vi "raptor.vi"(11 "Raptor Parameters":T1={"Vertical Search Range"=20, "Template Width"=180, "Template Height"=100, "Correlation Threshold"=0.5, "Surface Morph Size"=10, "En Face Width"=400, "En Face Height"=600, "En Face Depth"=15, "Aspect Ratio"=1.1, "Continous Scan"=FALSE, "Num En Face Reviews"=10, "Fluoresence Channel"=TRUE, "Track Depth"=TRUE, "Auto Expand"=TRUE, "Show Raptor Window"=TRUE, "Surface Threshold"=2, "Gaussian Filter Size"=1.5, "Mean Filter Size"=5.0}) -> ()   [LabVIEW 2016]
doc: "Main vi for Raptor OCT volume assembly system.\nMike Hughes, Applied Optics Group, University of Kent"
uses:
  typedef/raptor_parameters.ctl
  typedef/raptor_state.ctl
  <vilib>/vision/Image Controls.llb/IMAQ Image.ctl
  typedef/build_record.ctl
  typedef/raptor_states.ctl
  typedef/raptor_message.ctl
  typedef/raptor_image.ctl
  globals/Channel 1 Image Ring.vi
  globals/Channel 2 Image Ring.vi
  <vilib>/vision/NI_Vision_Development_Module.lvlib
  <vilib>/Analysis/NI_AALPro.lvlib
panel:
  out "B-scan Processed":i64=1000
  out "Surface Position":cluster{i32[], i32[]}(graph)={[2, 3, 4, 5, 6, 7, 8, 9, 11, 12, 13, 14, 15, 16, 17, 18, 19, 20, 21, 22, 23, 24, 25, 26, 28, 30, 40, 42, 45, 48, 51, 54, 56, 58, 60, 61, 63, 65, 67, 69, 71, 74, 76, 78, 80, 82, 84, 85, 87, 89, 91, 93, 95, 97, 99, 102, 104, 106, 108, 110, 112, 114, 117, 120, 123, 133, 137, 140, 143, 146, 149, 153, 157, 168, 171, 174, 177, 181, 186, 195, 198, 201, 205, 229, 233, 236, 238, 240, 243, 245, 249, 253, 259, 264, 268, 273, 276, 279, 282, 300, 302, 305, 307, 309, 311, 314, 321, 326, 329, 331, 333, 335, 336, 338, 340, 342, 344, 348, 354, 358, 361, 364, 366, 368, 370, 372, 374, 377, 380, 386, 390, 393, 396, 400, 405, 408, 410, 412, 414, 416, 417, 418, 419, 420, 421, 423, 425, 427, 429, 431, 434, 438, 441, 443, 445, 447, 448, 449, 450, 451, 452, 453, 454, 455, 456, 457, 458, 459, 461, 463, 465, 469, 484, 488, 490, 493, 495, 497, 499, 502, 506, 511, 515, 517, 519, 521, 522, 524, 526, 528, 537, 539, 541, 544, 549, 551, 553, 554, 556, 558, 560, 562, 564, 567, 569, 571, 573, 575, 577, 579, 581, 585, 594, 599, 602, 605, 607, 609, 611, 613, 616, 620, 625, 629, 634, 640, 644, 651, 653, 655, 661, 665, 673, 677, 681, 684, 687, 695, 700, 702, 704, 705, 707, 709, 711, 714, 718, 723, 726, 731, 734, 737, 742, 750, 753, 767, 780, 784, 801, 804, 806, 808, 810, 812, 814, 816, 818, 820, 823, 826, 828, 830, 832, 834, 836, 840, 844, 847, 850, 852, 854, 856, 858, 860, 864, 879, 883, 886, 888, 890, 892, 894, 896, 900, 903, 918, 920, 923, 925, 927, 929, 931, 933, 938, 949, 951, 953, 955, 958, 961, 964, 967, 970, 973, 977, 983, 988, 991, 994, 996, 999], [125, 124, 124, 124, 124, 124, 124, 125, 125, 125, 125, 125, 125, 126, 126, 126, 126, 126, 126, 125, 125, 125, 125, 125, 125, 125, 125, 125, 125, 125, 125, 122, 122, 122, 122, 122, 122, 122, 122, 122, 122, 122, 122, 120, 120, 120, 120, 120, 120, 125, 125, 125, 125, 125, 125, 130, 130, 130, 130, 130, 130, 132, 132, 132, 132, 132, 132, 138, 138, 138, 138, 138, 138, 144, 144, 144, 144, 144, 144, 154, 154, 154, 154, 154, 154, 157, 157, 157, 157, 157, 157, 166, 166, 166, 166, 166, 166, 168, 168, 168, 168, 168, 168, 165, 165, 165, 165, 165, 165, 177, 177, 177, 177, 177, 177, 180, 180, 180, 180, 180, 180, 176, 176, 176, 176, 176, 176, 175, 175, 175, 175, 175, 175, 176, 176, 176, 176, 176, 176, 173, 173, 173, 173, 173, 173, 173, 173, 173, 173, 173, 173, 169, 169, 169, 169, 169, 169, 163, 163, 163, 163, 163, 163, 163, 163, 163, 163, 163, 163, 160, 160, 160, 160, 160, 160, 158, 158, 158, 158, 158, 158, 165, 165, 165, 165, 165, 165, 162, 162, 162, 162, 162, 162, 158, 158, 158, 158, 158, 158, 161, 161, 161, 161, 161, 161, 160, 160, 160, 160, 160, 160, 160, 160, 160, 160, 160, 160, 162, 162, 162, 162, 162, 162, 164, 164, 164, 164, 164, 164, 172, 172, 172, 172, 172, 172, 170, 170, 170, 170, 170, 170, 176, 176, 176, 176, 176, 176, 185, 185, 185, 185, 185, 185, 188, 188, 188, 188, 188, 188, 209, 209, 209, 209, 209, 209, 214, 214, 214, 214, 214, 214, 208, 208, 208, 208, 208, 208, 201, 201, 201, 201, 201, 201, 197, 197, 197, 197, 197, 197, 195, 195, 195, 195, 195, 195, 196, 196, 196, 196, 196, 196, 203, 203, 203, 203, 203, 203, 209, 209, 209, 209, 209, 209, 207, 207, 207, 207, 207, 207, 207, 207]}
  out "Lateral Position":cluster{i32[], i32[]}(graph)={[2, 3, 4, 5, 6, 7, 8, 9, 11, 12, 13, 14, 15, 16, 17, 18, 19, 20, 21, 22, 23, 24, 25, 26, 28, 30, 40, 42, 45, 48, 51, 54, 56, 58, 60, 61, 63, 65, 67, 69, 71, 74, 76, 78, 80, 82, 84, 85, 87, 89, 91, 93, 95, 97, 99, 102, 104, 106, 108, 110, 112, 114, 117, 120, 123, 133, 137, 140, 143, 146, 149, 153, 157, 168, 171, 174, 177, 181, 186, 195, 198, 201, 205, 229, 233, 236, 238, 240, 243, 245, 249, 253, 259, 264, 268, 273, 276, 279, 282, 300, 302, 305, 307, 309, 311, 314, 321, 326, 329, 331, 333, 335, 336, 338, 340, 342, 344, 348, 354, 358, 361, 364, 366, 368, 370, 372, 374, 377, 380, 386, 390, 393, 396, 400, 405, 408, 410, 412, 414, 416, 417, 418, 419, 420, 421, 423, 425, 427, 429, 431, 434, 438, 441, 443, 445, 447, 448, 449, 450, 451, 452, 453, 454, 455, 456, 457, 458, 459, 461, 463, 465, 469, 484, 488, 490, 493, 495, 497, 499, 502, 506, 511, 515, 517, 519, 521, 522, 524, 526, 528, 537, 539, 541, 544, 549, 551, 553, 554, 556, 558, 560, 562, 564, 567, 569, 571, 573, 575, 577, 579, 581, 585, 594, 599, 602, 605, 607, 609, 611, 613, 616, 620, 625, 629, 634, 640, 644, 651, 653, 655, 661, 665, 673, 677, 681, 684, 687, 695, 700, 702, 704, 705, 707, 709, 711, 714, 718, 723, 726, 731, 734, 737, 742, 750, 753, 767, 780, 784, 801, 804, 806, 808, 810, 812, 814, 816, 818, 820, 823, 826, 828, 830, 832, 834, 836, 840, 844, 847, 850, 852, 854, 856, 858, 860, 864, 879, 883, 886, 888, 890, 892, 894, 896, 900, 903, 918, 920, 923, 925, 927, 929, 931, 933, 938, 949, 951, 953, 955, 958, 961, 964, 967, 970, 973, 977, 983, 988, 991, 994, 996, 999], [-2, -3, -3, -4, -4, -4, -6, -5, -7, -7, -9, -10, -2, 7, 8, 8, 4, 7, 6, 5, 12, 15, 15, 15, 17, 16, 18, 18, 17, 17, 20, 14, 13, 13, 14, 15, 8, 8, 8, 8, 10, 13, 15, 15, 14, 17, 18, 17, 14, 15, 14, 14, 13, 12, 11, 11, 12, 12, 12, 11, 12, 11, 10, 8, 7, 4, 4, 3, 2, 3, 4, 4, 1, -4, -4, -4, -5, -7, -10, -10, -11, -13, -17, -26, -24, -25, -27, -29, -31, -31, -32, -32, -32, -33, -34, -32, -31, -30, -30, -31, -31, -30, -30, -29, -29, -28, -30, -30, -29, -27, -28, -28, -27, -27, -27, -26, -27, -28, -31, -32, -32, -32, -32, -32, -31, -32, -34, -35, -37, -40, -42, -44, -47, -49, -51, -50, -49, -48, -43, -45, -43, -43, -42, -43, -42, -41, -38, -35, -35, -34, -34, -31, -31, -32, -30, -33, -32, -29, -27, -26, -22, -19, -17, -14, -12, -9, -7, -6, -3, -1, 0, 0, -8, -7, -7, -7, -7, -7, -7, -6, -5, -2, 0, 2, 6, 8, 10, 13, 16, 19, 20, 21, 21, 23, 28, 31, 34, 36, 37, 40, 41, 42, 44, 45, 47, 47, 47, 48, 48, 47, 46, 43, 33, 27, 24, 28, 26, 24, 24, 23, 22, 19, 15, 12, 6, 0, -2, -4, -5, -8, -14, -22, -32, -40, -48, -52, -56, -66, -71, -71, -69, -69, -70, -71, -72, -73, -74, -77, -79, -84, -88, -92, -99, -107, -109, -112, -122, -127, -132, -133, -134, -134, -133, -133, -133, -132, -132, -132, -131, -130, -130, -129, -127, -127, -127, -124, -123, -122, -120, -119, -119, -119, -118, -116, -116, -116, -118, -119, -118, -118, -120, -120, -128, -138, -136, -136, -137, -137, -137, -134, -133, -133, -132, -128, -119, -117, -107, -106, -104, -101, -98, -97, -96, -96, -97, -97, -95, -94, -93, -92, -93]}
  out "Velocity":cluster{i32[], dbl[]}(graph)={[2, 3, 4, 5, 6, 7, 8, 9, 11, 12, 13, 14, 15, 16, 17, 18, 19, 20, 21, 22, 23, 24, 25, 26, 28, 30, 40, 42, 45, 48, 51, 54, 56, 58, 60, 61, 63, 65, 67, 69, 71, 74, 76, 78, 80, 82, 84, 85, 87, 89, 91, 93, 95, 97, 99, 102, 104, 106, 108, 110, 112, 114, 117, 120, 123, 133, 137, 140, 143, 146, 149, 153, 157, 168, 171, 174, 177, 181, 186, 195, 198, 201, 205, 229, 233, 236, 238, 240, 243, 245, 249, 253, 259, 264, 268, 273, 276, 279, 282, 300, 302, 305, 307, 309, 311, 314, 321, 326, 329, 331, 333, 335, 336, 338, 340, 342, 344, 348, 354, 358, 361, 364, 366, 368, 370, 372, 374, 377, 380, 386, 390, 393, 396, 400, 405, 408, 410, 412, 414, 416, 417, 418, 419, 420, 421, 423, 425, 427, 429, 431, 434, 438, 441, 443, 445, 447, 448, 449, 450, 451, 452, 453, 454, 455, 456, 457, 458, 459, 461, 463, 465, 469, 484, 488, 490, 493, 495, 497, 499, 502, 506, 511, 515, 517, 519, 521, 522, 524, 526, 528, 537, 539, 541, 544, 549, 551, 553, 554, 556, 558, 560, 562, 564, 567, 569, 571, 573, 575, 577, 579, 581, 585, 594, 599, 602, 605, 607, 609, 611, 613, 616, 620, 625, 629, 634, 640, 644, 651, 653, 655, 661, 665, 673, 677, 681, 684, 687, 695, 700, 702, 704, 705, 707, 709, 711, 714, 718, 723, 726, 731, 734, 737, 742, 750, 753, 767, 780, 784, 801, 804, 806, 808, 810, 812, 814, 816, 818, 820, 823, 826, 828, 830, 832, 834, 836, 840, 844, 847, 850, 852, 854, 856, 858, 860, 864, 879, 883, 886, 888, 890, 892, 894, 896, 900, 903, 918, 920, 923, 925, 927, 929, 931, 933, 938, 949, 951, 953, 955, 958, 961, 964, 967, 970, 973, 977, 983, 988, 991, 994, 996, 999], [1.143797746307766, 1.3333396872995098, 1.2487410409443742, 1.3775792507370008, 1.35235696427408, 1.0958240904186254, 1.2676013637456374, 0.6145742688419122, 1.3642108384733156, 1.3291502502216916, 1.21069468600585, 1.5066752009600175, 1.3185798676443576, 1.3061268806293196, 1.4800464305533785, 1.2598267602292732, 1.27380930432652, 1.4864245752223852, 1.2430004595317607, 1.136871930852872, 1.3945928479025902, 1.1757526231458468, 1.2501477187489025, 0.6448381290998326, 0.6552015477217997, 0.11509297005760484, 0.5254258313307278, 0.42124218869463326, 0.35170783035527775, 0.4004315790880685, 0.5002809800482385, 0.7271073646002897, 0.5999592851493059, 0.540690558294546, 1.1801607790090474, 0.5119097105437318, 0.7113094368879718, 0.6284082783175837, 0.5497602971784958, 0.5726895632481627, 0.37986841633129165, 0.6592129730625476, 0.6349057739318787, 0.6777422202596586, 0.6299509242395064, 0.6899735269478533, 1.38105293249968, 0.5606455662414541, 0.6772054230606959, 0.5924100969444757, 0.7149037988988747, 0.5767179504655686, 0.5649603741065153, 0.5828407642135458, 0.33920879059135844, 0.5645755532640904, 0.5238204542972316, 0.6266600518224832, 0.695284771260091, 0.5880308825842286, 0.5231041763729385, 0.411874856446439, 0.4338825160604348, 0.3865914932469118, 0.1131585044335421, 0.2920781860842516, 0.3850511052033991, 0.3612918342022492, 0.4038055913676509, 0.4144135372286516, 0.3378572765322262, 0.2980472612185606, 0.09217265620143311, 0.35421388723830916, 0.3391541864077577, 0.4210005189327873, 0.34697024742461174, 0.2222414620799441, 0.1193934466280525, 0.41120661977345413, 0.3400793994587875, 0.31426638667428675, 0.047587903067617066, 0.2770631920263342, 0.38516412890611046, 0.6649694993911732, 0.5728710397311542, 0.3506214247140595, 0.5848076270081521, 0.2570561563150278, 0.30361075452375375, 0.1742645462204123, 0.223343307545586, 0.3100195925244551, 0.2074844375532454, 0.37988813162246887, 0.4144806925940141, 0.41332167059800895, 0.056941045416284856, 0.5698218136390614, 0.3520130034487336, 0.6432387277552128, 0.5833582043546514, 0.556857352931591, 0.3662981901452101, 0.16037251779007075, 0.21687316163296827, 0.3999701574821297, 0.6353717491435529, 0.6454379977704356, 0.615708336426717, 1.41792494969707, 0.537393274100483, 0.7700097401475798, 0.7593871184623432, 0.5687041954401564, 0.26298300241046013, 0.20434354639333707, 0.25948634210038984, 0.34419524518070227, 0.40925827871997716, 0.5378841781340442, 0.6769555720217142, 0.6349141889837975, 0.6834463670259239, 0.7025641215978294, 0.4504390062285957, 0.44386269848744375, 0.19099573410844067, 0.301540032968191, 0.3355780928472318, 0.3445169234861601, 0.29506141873143077, 0.20505526192536022, 0.37073524038941247, 0.5221774899519338, 0.5469741896295042, 0.7036983466543694, 0.7092045906659568, 1.5395407544538646, 1.1129889550086198, 1.0662046005039005, 1.1679340457582295, 1.0428105476236473, 0.5829152768189518, 0.7207799665048271, 0.7454220022900797, 0.7578460704893974, 0.6178007921722288, 0.39904061516545886, 0.3750096579891553, 0.3739159454440689, 0.5976008979796122, 0.6693660164052238, 0.6315608514418974, 1.4939995236566106, 1.1338784343578556, 1.3314623582386393, 1.3580510315534005, 1.4815643675333285, 1.2988829886909206, 1.2345614429309268, 1.2934510994433377, 1.3301345167302814, 1.4167367228316123, 1.2165168813930995, 1.2019487859022253, 0.5410110137929889, 0.7152002307851674, 0.7115865730776564, 0.32031429412027806, 0.07680639720443082, 0.2538304248879253, 0.6478327571011689, 0.3485830083671217, 0.6103184454642819, 0.6411873103800232, 0.6711137093424853, 0.43162702301911515, 0.30315198727144976, 0.248601818682715, 0.3034164901028119, 0.5135004026713286, 0.5329906512462365, 0.6717381863722649, 1.3015826219782702, 0.5077458404876318, 0.6396927938855128, 0.6800806248882034, 0.1734987926362407, 0.637736803565148, 0.5228090310254856, 0.36254771299448224, 0.20015119481035654, 0.5243991505889207, 0.5883754615132863, 1.3287278063623198, 0.5046369732664049, 0.8205042689283863, 0.7427053274034519, 0.7232804846763172, 0.6287228406956029, 0.4099021437070359, 0.6143602797934619, 0.7841152365157958, 0.5459109583971835, 0.5571037443792013, 0.7250054234943955, 0.6720045824988568, 0.7324927913288382, 0.27352657827006854, 0.11139123112524134, 0.21315769068017892, 0.3630512774958517, 0.3985447957883489, 0.7379760266761712, 0.5178926074628747, 0.6114472213145665, 0.6575786152357235, 0.40499495419995474, 0.3061391384268032, 0.20131656355332794, 0.2756359455730823, 0.2083165585365504, 0.20200339125056965, 0.2742044661408461, 0.1490228595501116, 0.5632965165147921, 0.5340470481770991, 0.2125127305130901, 0.3367649025713827, 0.15223269989429117, 0.39141997685846663, 0.2964256363237714, 0.36271684609005866, 0.36996756484547977, 0.14890238150787583, 0.21362297674623185, 0.577447744155924, 0.6322065874120464, 1.7735416128234527, 0.5144967831712401, 0.7446067300050981, 0.577768254182741, 0.35979743501712197, 0.25930498945797853, 0.22741754812420986, 0.38772812696105385, 0.24233165924969474, 0.374074933893613, 0.4231664162601074, 0.22921343478040007, 0.13638231132950795, 0.3333656987138862, 0.07756488579990443, 0.08279503777441793, 0.2641964865383801, 0.0624360565039626, 0.3904523790292849, 0.7236046317833084, 0.5724041571099163, 0.508801563641412, 0.5692508174696873, 0.5521987720388553, 0.5188437616401143, 0.5018066245215063, 0.5948609972965777, 0.3576148381717812, 0.3890957023690013, 0.6521927564387369, 0.7140931457916087, 0.672299826075009, 0.6993435415185927, 0.7103653224813742, 0.26811849860305903, 0.32331542311737277, 0.3941850971730236, 0.42233083440496555, 0.6884612996210246, 0.576079583394164, 0.6187361954646837, 0.5957777118096641, 0.5668641641399372, 0.3319985734829252, 0.07061994988983814, 0.29629732710784745, 0.3837685541892542, 0.6678492438425538, 0.560674744259874, 0.5663073112889818, 0.7681102904861878, 0.5559444123228814, 0.2506641792895014, 0.455697393798198, 0.0731179626490377, 0.5727103819153584, 0.34743439462532716, 0.5134413085650353, 0.5115506974044023, 0.7237801217250202, 0.731537263007918, 0.6083882190824177, 0.22547899949164282, 0.09154896569808366, 0.6666134315908854, 0.6692380584223405, 0.7859074862502353, 0.40622478823765285, 0.4012636506114792, 0.3500423294645012, 0.37585640414677374, 0.43256742703814044, 0.41046228950735647, 0.26500064441419924, 0.2073145191037447, 0.21294437480002826, 0.4009521682930483, 0.38096792810336483, 0.690240158669222, 0.44981325347101175, inf]}
  in  "Track Surface":bool=TRUE
  out "Frame Step":dbl=1.3415904319230465 format="%#.2g"
  in  "Enface Display Depth":i64=15
  in  "Save En Face From Volume":bool
  in  "Save En Face Button":bool
  in  "Save Folder":path
  in  "Save Volume Button":bool
  out "Fluorescence Review":T2(plugin-control)
  out "Corrected Fluorescence":T2(plugin-control)
  out "Running":bool
  in  "Current Volume Review Selector":i64(slide)=20 scale=0.0..600.0
  in  "En Face Review Selector":i8(slide) scale=0.0..10.0
  out "Current Volume En Face Review":T2(plugin-control)
  out "En Face Review":T2(plugin-control)
  out "Frame Lag":i32
  out "Frame Rate":dbl=2.119876203085889e-05 format="%#.0f"
  out "Y Shift":i32=-2
  out "X Shift":i32=-1
  out "En Face Line":dbl=429.83712890006 format="%#.2f"
  out "Y Position":i32=-133
  out "X Position":i32=-92
  out "Decorrelated":bool
  out "Correlation":dbl=0.944969845185697 format="%#_2g"
  out "Corrected En Face":T2(plugin-control)
  in  "New Scan Button":bool
  in  "Start Button":bool
  in  "Stop Button":bool
  in  "Shutdown Button":bool
  out "Current B Scan":T2(plugin-control)
  # "Monitor"
  # "Applied Optics Group"
  # "Review Image \nNo. to Display"
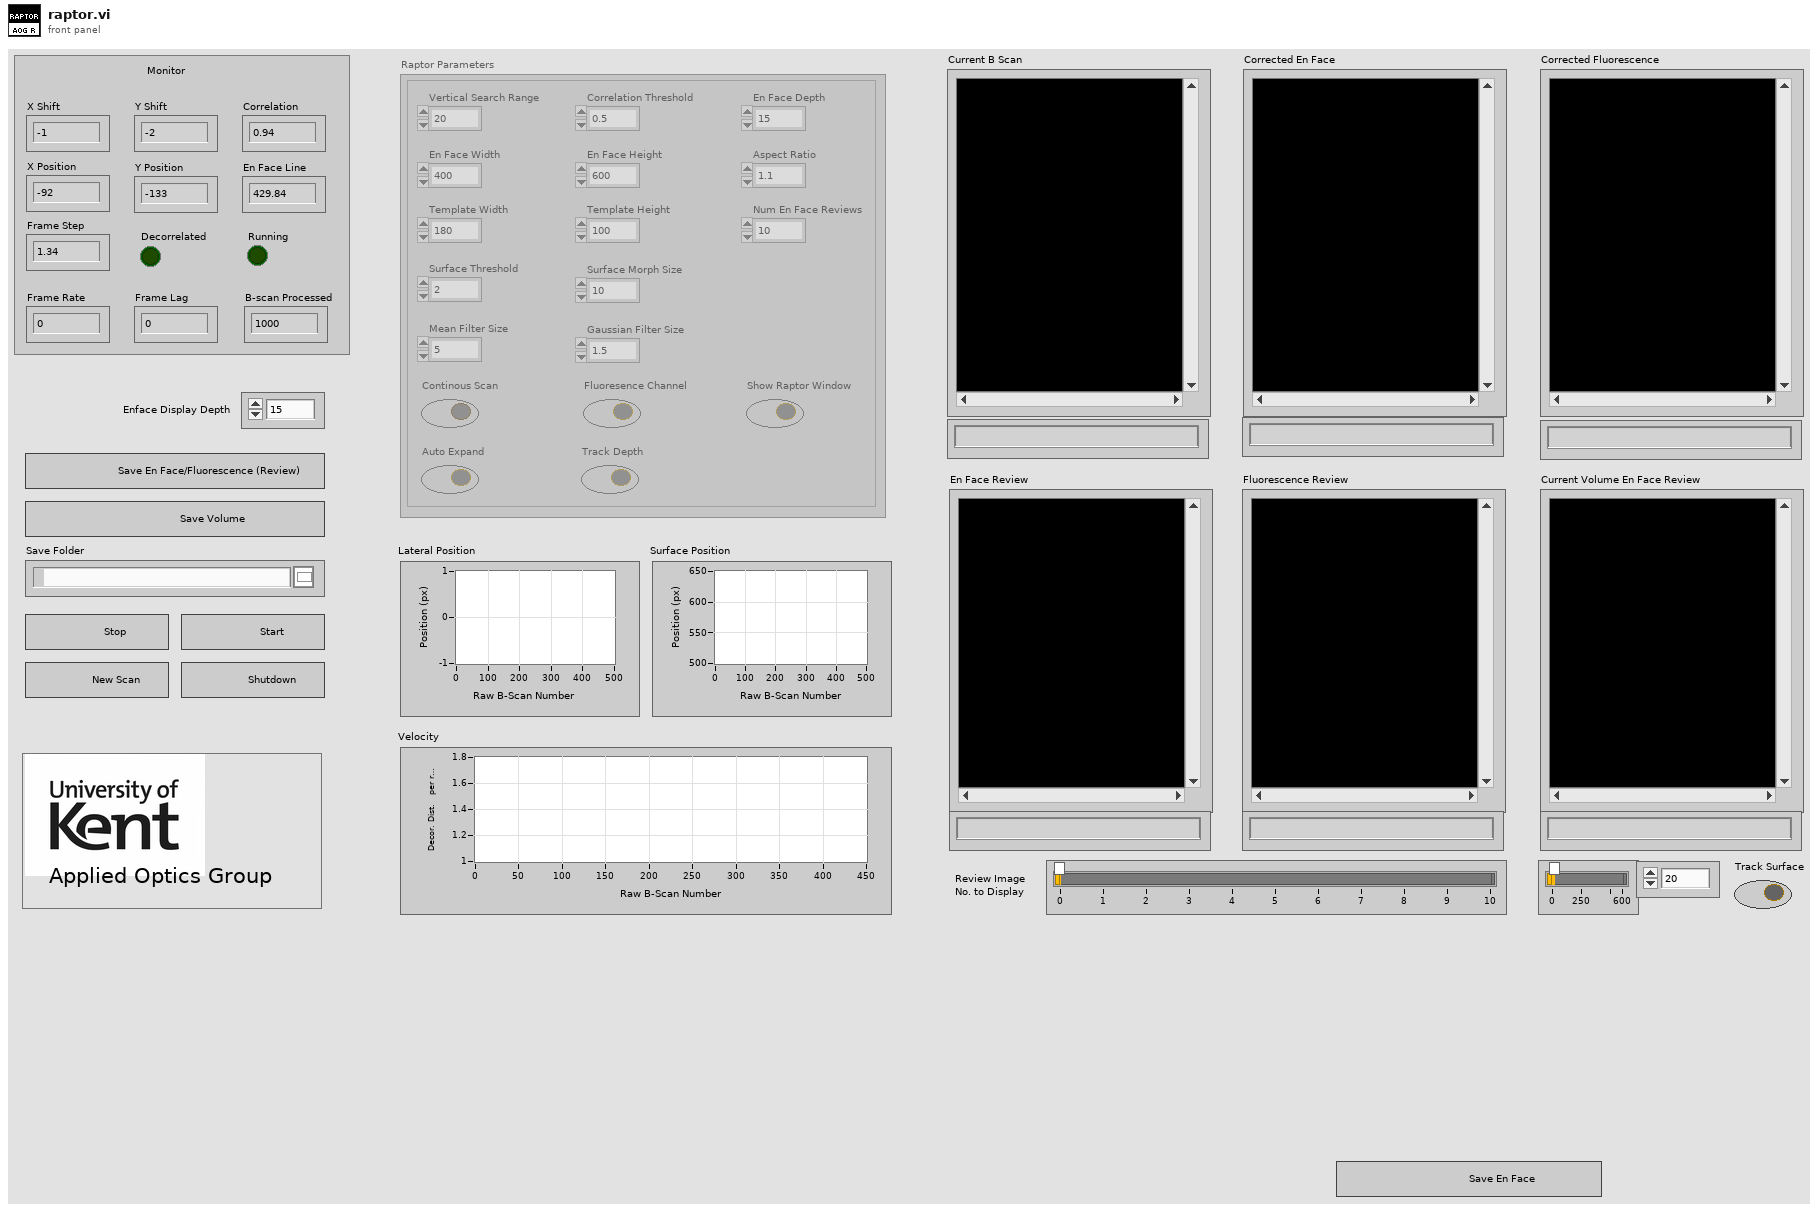
[diagram p1: front panel]
types:
  T1 = typedef "raptor_parameters.ctl" = cluster{"Vertical Search Range":i32, "Template Width":i32, "Template Height":i32, "Correlation Threshold":dbl, "Surface Morph Size":i32, "En Face Width":i32, "En Face Height":i32, "En Face Depth":i32, "Aspect Ratio":dbl, "Continous Scan":bool, "Num En Face Reviews":i32, "Fluoresence Channel":bool, "Track Depth":bool, "Auto Expand":bool, "Show Raptor Window":bool, "Surface Threshold":i32, "Gaussian Filter Size":dbl, "Mean Filter Size":dbl}
  T2 = typedef "IMAQ Image.ctl" = refnum<image>
  T3 = typedef "raptor_states.ctl" = enum16{"--- INIT ---", "initialise", "constants", "create images", "--- DATA FUNCTIONS ---", "surface find", "shift find", "check correlation", "build corrected OCT", "build corrected Fluor", "prepare reference image", "record corrected", "auto expand", "generate plots", "--- GUI HANDING ---", "update images", "update parameters", "save volume en face", "set volume review", "--- PROCESS FLOW ---", "wait", "process image", "increment linepos", "handle decorrelation", "start", "stop", "new scan", "end scan", "shutdown", "check stable scan", "--- LOAD AND SAVE ---", "save all", "save en face", "save fluorescence", "set en face review", "save volume"}
  T4 = typedef "raptor_image.ctl" = cluster{"Data":variant, "Image":T2}
  T5 = typedef "raptor_message.ctl" = cluster{"Message":enum16{"start", "stop", "initialise", "shutdown", "end scan", "new scan", "set depth"}, "Data":variant}
  T6 = typedef "raptor_state.ctl" = cluster{"Running":bool, "Template":T2, "Current Image":T2, "Ref Cropped":T2, "Ref Image":T2, "Current Depth":i32, "ROI Width":i32, "ROI Height":i32, "Vertical Search Range":i32, "Correlation":dbl, "Y Shift":i32, "X Shift":i32, "En Face":T2, "X Pos":i32, "Y Pos":i32, "En Face Depth":i32, "En Face Width":i32, "En Face Height":i32, "Decorrelated":bool, "Correlation Thresh":dbl, "Surface Morph SIze":dbl, "Corrected Linepos":dbl, "Last Line":dbl, "Aspect Ratio":dbl, "Continuous Scan":bool, "En Face Review":T2[], "En Face Counter":i64, "Num En Face Reviews":i32, "B Scan Counter":i64, "Volume En Face":T2, "Current Scan Images":T2[], "Line Counter":i32, "Fluorescence Channel":bool, "Fluorescence Line":T2, "Fluorescence Image":T2, "Fluorescence Review":T2[], "Track Surface":bool, "Min Lines for Review":i32, "Stability Length":i32, "Auto Expand":bool, "Image Type":T7, "Expand Step":i32, "Surface Threshold":dbl, "ROI  Vertical Offset":i32, "Current ROI":T2, "Reference ROI":T2, "Mean Filter Size":i32, "Gaussian Filter Size":dbl, "Build Record":T8[], "Temp Image":T2, "Reference Filtered":dbl[][], "Frame Step":dbl, "Volume Review Depth Shown":i64, "Surface Find Regularity":i32, "Image Display Regularity":i32}
  T7 = typedef "Image Type" = u32
  T8 = typedef "build_record.ctl" = cluster{"xPos":i32, "yPos":i32, "B-scan":i32, "Correlation":dbl, "Frame Step":dbl}
  T9 = enum16{"start", "stop", "initialise", "shutdown", "end scan", "new scan", "set depth"}
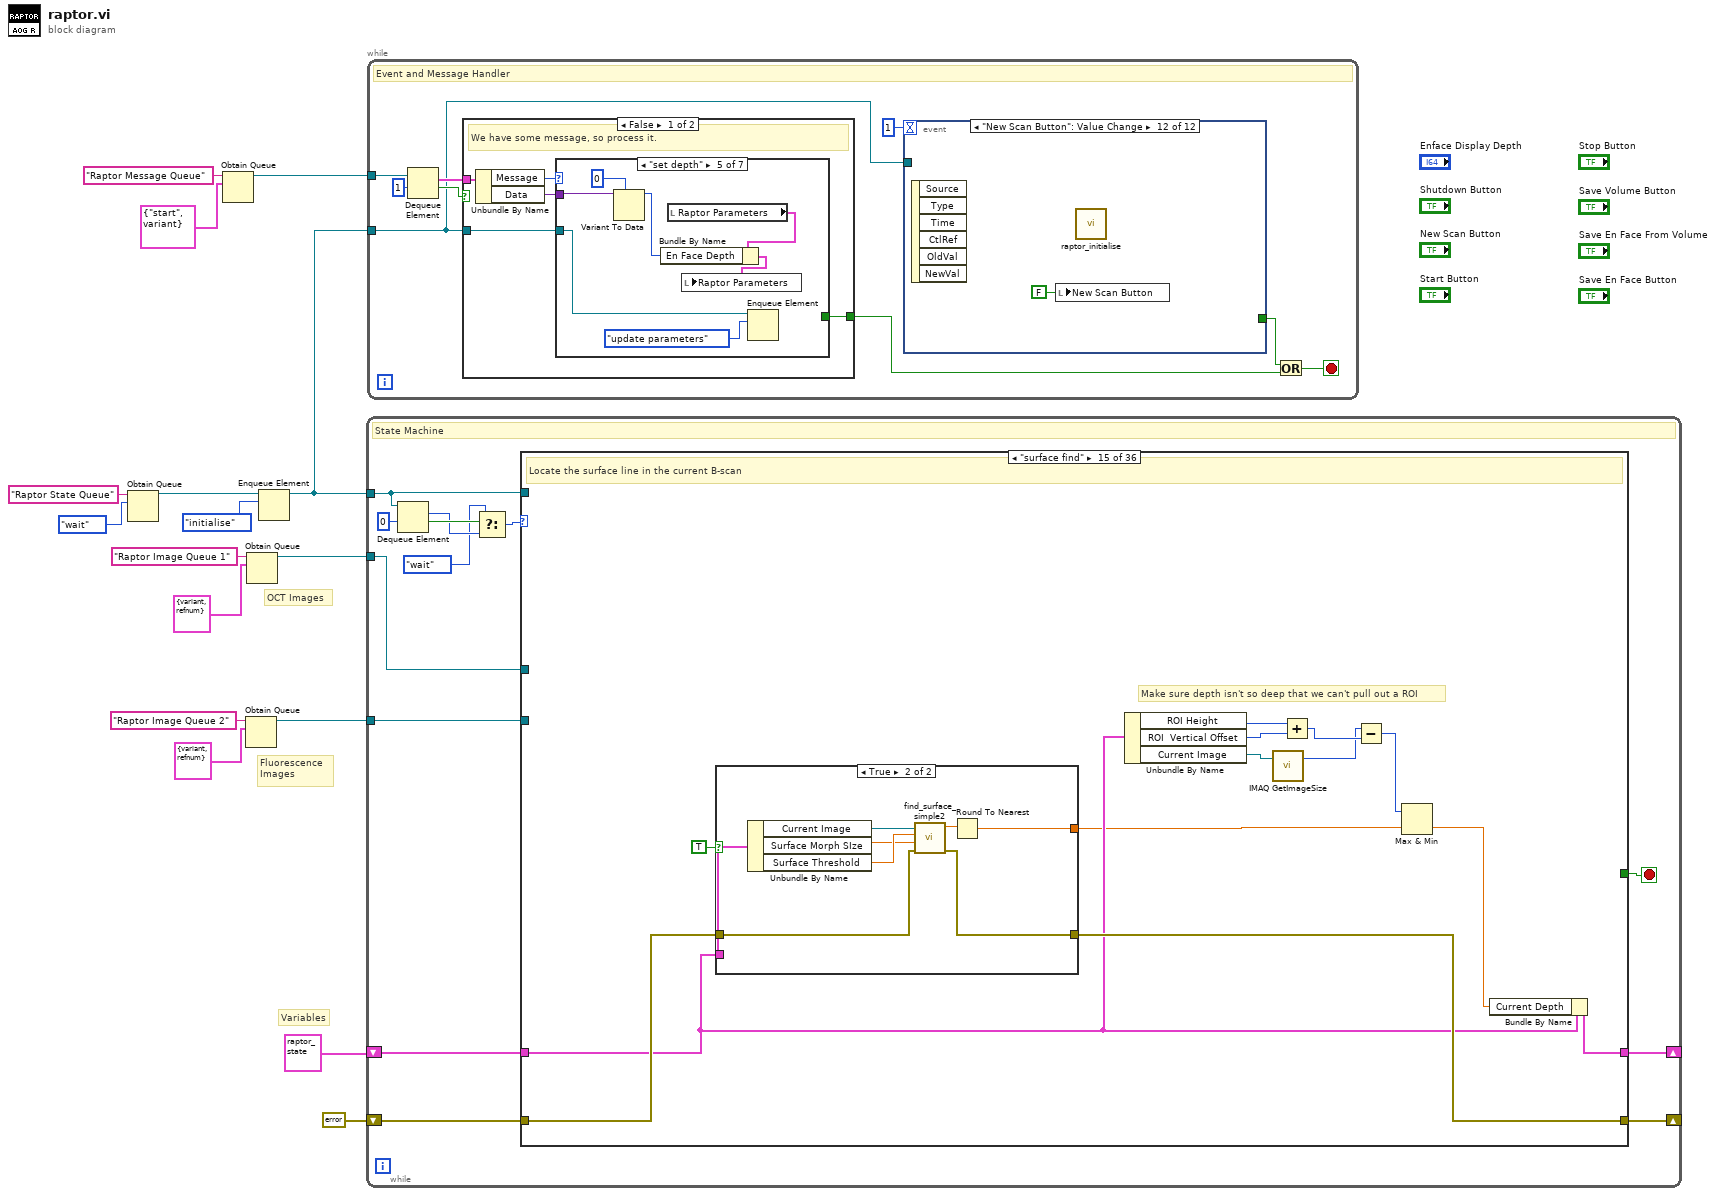
[diagram p0: block diagram]
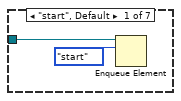
[diagram p2: hidden frame]
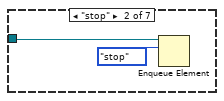
[diagram p3: hidden frame]
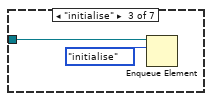
[diagram p4: hidden frame]
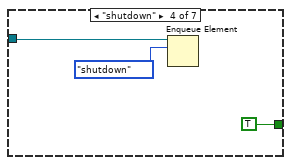
[diagram p5: hidden frame]
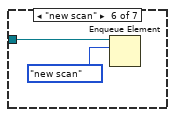
[diagram p6: hidden frame]
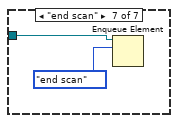
[diagram p7: hidden frame]
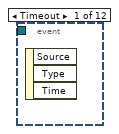
[diagram p9: hidden frame]
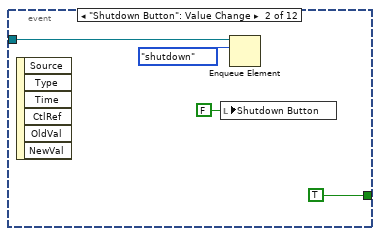
[diagram p10: hidden frame]
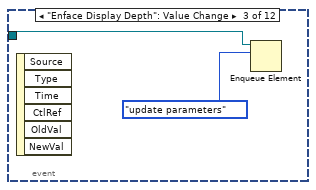
[diagram p11: hidden frame]
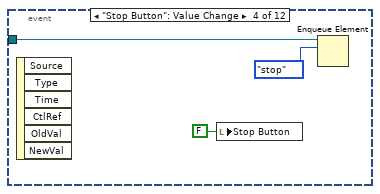
[diagram p12: hidden frame]
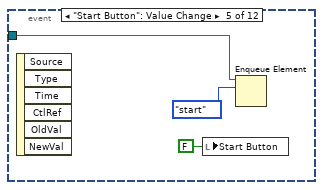
[diagram p13: hidden frame]
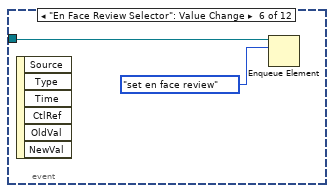
[diagram p14: hidden frame]
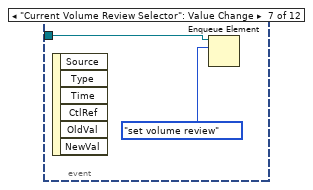
[diagram p15: hidden frame]
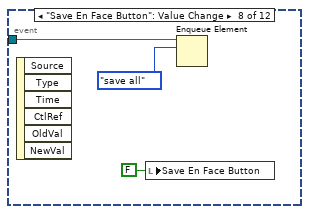
[diagram p16: hidden frame]
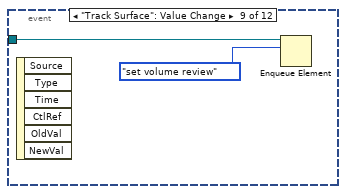
[diagram p17: hidden frame]
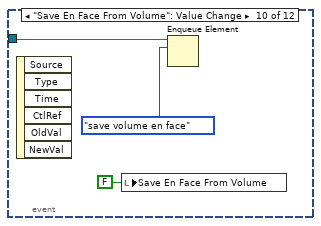
[diagram p18: hidden frame]
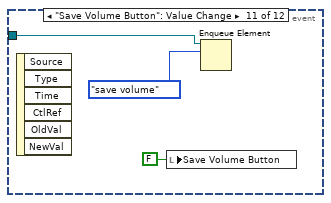
[diagram p19: hidden frame]
diagram:
  # "Fluorescence \nImages"
  # "OCT Images"
  # "Variables"
  n1 = Obtain Queue(name (unnamed)="Raptor State Queue", element data type=raptor_states."wait") -> (queue out=w5:refnum<queue>)  [unwired: 3 in, 2 out]
  n2 = Obtain Queue(name (unnamed)="Raptor Message Queue", element data type=T5 {"Message"=enum."start", "Data"=variant}) -> (queue out=w14:refnum<queue>)  [unwired: 3 in, 2 out]
  n3 = Obtain Queue(name (unnamed)="Raptor Image Queue 2", element data type=T4 {"Data"=variant, "Image"=refnum}) -> (queue out=w9:refnum<queue>)  [unwired: 3 in, 2 out]
  n4 = Obtain Queue(name (unnamed)="Raptor Image Queue 1", element data type=T4 {"Data"=variant, "Image"=refnum}) -> (queue out=w11:refnum<queue>)  [unwired: 3 in, 2 out]
  n5 = Enqueue Element(queue=w5, element=raptor_states."initialise") -> (queue out=w4:refnum<queue>)  [unwired: 2 in, 2 out]
  n6 = while {
    tunnel: w4 -> [w22]
    tunnel: w11 -> [w29]
    tunnel: w9 -> [w28]
    shift-right: [w24] -> _
    shift-left: T6 {"Running"=TRUE, "Template"=refnum, "Current Image"=refnum, "Ref Cropped"=refnum, "Ref Image"=refnum, "Current Depth"=0, "ROI Width"=0, "ROI Height"=0, "Vertical Search Range"=0, "Correlation"=0.0, "Y Shift"=0, "X Shift"=0, "En Face"=refnum, "X Pos"=0, "Y Pos"=0, "En Face Depth"=0, "En Face Width"=0, "En Face Height"=0, "Decorrelated"=FALSE, "Correlation Thresh"=0.0, "Surface Morph SIze"=0.0, "Corrected Linepos"=0.0, "Last Line"=0.0, "Aspect Ratio"=0.0, "Continuous Scan"=FALSE, "En Face Review"=[], "En Face Counter"=0, "Num En Face Reviews"=0, "B Scan Counter"=0, "Volume En Face"=refnum, "Current Scan Images"=[], "Line Counter"=0, "Fluorescence Channel"=FALSE, "Fluorescence Line"=refnum, "Fluorescence Image"=refnum, "Fluorescence Review"=[], "Track Surface"=FALSE, "Min Lines for Review"=0, "Stability Length"=0, "Auto Expand"=FALSE, "Image Type"=0, "Expand Step"=0, "Surface Threshold"=0.0, "ROI  Vertical Offset"=0, "Current ROI"=refnum, "Reference ROI"=refnum, "Mean Filter Size"=0, "Gaussian Filter Size"=0.0, "Build Record"=[], "Temp Image"=refnum, "Reference Filtered"=[], "Frame Step"=0.0, "Volume Review Depth Shown"=0, "Surface Find Regularity"=0, "Image Display Regularity"=0} -> [w23]
    shift-right: [w25] -> _
    shift-left: errorcluster {"status"=FALSE, "code"=0, "source"=""} ("error out") -> [w26]
    stop <- w27 stop-if-true
    # "State Machine"
    n7 = Dequeue Element(queue=w22, timeout in ms (-1)=0) -> (element=w19:T3, timed out?=w20:bool)  [unwired: 1 in, 2 out]
    n8 = Select(t=raptor_states."wait" ("element"), s=w20, f=w19) -> (s? t:f=w17:T3)
    n9 = case shown="\"surface find\"" w17 {
      tunnel: w22 -> [_ w45 _ _ _ w119 _ _ w153 _ w166 w218 w247 _ _ _ w343 _ _ _ _ w403 w452 _ _ w481 _ _ _ _ _ w549 _ _ _ _]
      tunnel: w23 -> [w30 w42 w77 w88 w115 w122 w130 w133 w140 w161 w169 w213 w251 w270 w280 w304 w325 w348 w371 w373 w387 w402 w447 w468 w477 w485 w494 w499 w523 w532 w544 w550 w558 w561 w573 w605]
      tunnel: w29 -> [_ _ _ _ _ w117 _ _ _ _ _ w233 _ _ _ _ _ _ _ _ _ _ _ _ _ _ _ _ _ _ _ _ _ _ _ _]
      tunnel: w28 -> [_ _ _ _ _ _ _ _ _ _ _ w223 _ _ _ _ _ _ _ _ _ _ _ _ _ _ _ _ _ _ _ _ _ _ _ _]
      tunnel: [_ _ _ _ _ _ _ _ _ TRUE _ _ _ _ _ _ _ _ _ _ _ _ _ _ _ _ _ _ _ _ _ _ _ _ _ _] -> w27
      tunnel: w26 -> [w31 w33 w71 w78 w114 w123 w127 w131 w137 _ w165 w210 w244 w271 w284 w305 w315 w352 _ w372 w388 w404 w454 w472 w478 w479 _ _ w519 w526 w543 w545 w551 w559 w572 w608]
      tunnel: [w31 w33 w71 w78 w114 w123 w127 w131 w137 _ w165 w210 w244 w271 w283 w305 w315 w353 _ w372 w388 w404 w454 w472 w478 w479 _ _ w519 w526 w543 w545 w551 w559 w570 w607] -> w25
      tunnel: [w30 w47 w76 w95 w115 w122 w128 w132 w146 w161 w181 w224 w251 w270 w281 w307 w332 w347 w371 w373 w400 w402 w451 w468 w477 w485 w493 w499 w523 w531 w544 w550 w558 w561 w573 w605] -> w24
      frame "--- INIT ---" {
      }
      frame "initialise" {
        w34 = cluster{dbl[], "dX/dt":dbl[]} {[], "dX/dt"=[]} ("Lateral Position")
        w51 = FALSE
        # "Clear graphs"
        # "Make sure buttons are unpressed"
        # "Copies values from\nthe parameters passed\nby the caller."
        # "Start up routines, initialise parameters in main cluster variable, check all buttons are unpressed, clear graphs."
        n10 = Enqueue Element(queue=w45, element=raptor_states."constants") -> (queue out=w44:refnum<queue>)  [unwired: 2 in, 2 out]
        n11 = Enqueue Element(queue=w44, element=raptor_states."create images") -> (queue out=w55:refnum<queue>)  [unwired: 2 in, 2 out]
        n12 = Unbundle By Name("Raptor Parameters") -> ("En Face Width"=w58:i32, "En Face Height"=w53:i32, "Num En Face Reviews"=w54:i32)
        n13 = Unbundle By Name("Raptor Parameters") -> ("Show Raptor Window"=w41:bool)
        n14 = Enqueue Element(queue=w55, element=raptor_states."new scan") -> ()  [unwired: 2 in, 3 out]
        n15 = Unbundle By Name("Raptor Parameters") -> ("Fluoresence Channel"=w52:bool, "Track Depth"=w49:bool, "Auto Expand"=w43:bool, "Aspect Ratio"=w35:dbl)
        n16 = Unbundle By Name("Raptor Parameters") -> ("Gaussian Filter Size"=w39:dbl, "Mean Filter Size"=w38:dbl, "Surface Threshold"=w40:i32, "Vertical Search Range"=w63:i32, "Template Width"=w62:i32, "Template Height"=w61:i32, "Correlation Threshold"=w60:dbl, "Surface Morph Size"=w59:i32, "En Face Depth"=w50:i32, "Continous Scan"=w48:bool)
        n17 = case shown="True" w41 {
          frame False {
            n18 = control-ref of="This VI"() -> (w65:refnum<vi>)
            n19 = invoke class="VI" method="FP.Close"(reference=w65) -> (reference out=w66:refnum<vi>)  [unwired: 2 in, 2 out]
            n20 = Close Reference(reference=w66) -> ()  [unwired: 1 in, 1 out]
          }
          frame True {
            n21 = control-ref of="This VI"() -> (w68:refnum<vi>)
            n22 = invoke class="VI" method="FP.Open"(reference=w68) -> (reference out=w67:refnum<vi>)  [unwired: 4 in, 4 out]
            n23 = Close Reference(reference=w67) -> ()  [unwired: 1 in, 1 out]
          }
        }
        n24 = property on="En Face Review Selector" class="Slide (strict)"("Scale.Maximum"=w54) -> ()  [unwired: 2 in, 2 out]
        n25 = Initialize Array(T8 {"xPos"=0, "yPos"=0, "B-scan"=0, "Correlation"=0.0, "Frame Step"=0.0} ("Cluster"), w53) -> (w36:T8[])
        n26 = local write "Enface Display Depth"(w50) -> ()
        n27 = Bundle By Name(cluster=w42, "Gaussian Filter Size"=w39, "Mean Filter Size"=w38, "Surface Threshold"=w40, "Vertical Search Range"=w63, "ROI Width"=w62, "ROI Height"=w61, "Correlation Thresh"=w60, "Surface Morph SIze"=w59, "En Face Depth"=w50, "Continuous Scan"=w48, "En Face Width"=w58, "En Face Height"=w53, "Corrected Linepos"=0.0, "Num En Face Reviews"=w54, "Build Record"=w36, "Fluorescence Channel"=w52, "Track Surface"=w49, "Auto Expand"=w43, "Aspect Ratio"=w35) -> (w47:T6)
        n28 = local write "Stop Button"(w51) -> ()
        n29 = local write "Save En Face From Volume"(w51) -> ()
        n30 = local write "Start Button"(w51) -> ()
        n31 = local write "New Scan Button"(w51) -> ()
        n32 = local write "Shutdown Button"(w51) -> ()
        n33 = local write "Save Volume Button"(w51) -> ()
        n34 = local write "Save En Face Button"(w51) -> ()
        n35 = local write "Lateral Position"(w34) -> ()
        n36 = local write "Velocity"(w34) -> ()
        n37 = local write "Surface Position"(w34) -> ()
      }
      frame "constants" {
        w72 = T7 0 items=["Grayscale (U8)", "Grayscale (I16)", "Grayscale (SGL)", "Complex (CSG)", "RGB (U32)", "HSL (U32)", "RGB (U64)", "Grayscale (U16)"] ("Image Type")
        # "Set hard-coded constants."
        n38 = Bundle By Name(cluster=w77, "Stability Length"=10, "Min Lines for Review"=20, "Image Type"=w72, "Expand Step"=40, "Surface Find Regularity"=6, "Image Display Regularity"=20) -> (w76:T6)
      }
      frame "create images" {
        # "Creates all IMAQ images"
        n39 = Unbundle By Name(w88) -> ("Num En Face Reviews"=w91:i32)
        n40 = Unbundle By Name(w88) -> ("En Face Height"=w99:i32)
        n41 = Unbundle By Name(w88) -> ("Image Type"=w80:T7)
        n42 = call "create_image_array.vi"("Prefix"="Raptor Volume", "Image Type"=w80, "Num Images"=w99) -> ("Image Array"=w97:T2[])  [unwired: 7 in, 1 out]
        n43 = call "IMAQ Create"("Image Name"="Raptor Ref Image", "Image Type"=w80) -> ("New Image"=w108:T2)  [unwired: 3 in, 1 out]
        n44 = call "IMAQ Create"("Image Name"="Raptor Ref Cropped", "Image Type"=w80) -> ("New Image"=w107:T2)  [unwired: 3 in, 1 out]
        n45 = call "IMAQ Create"("Image Name"="Raptor Current Image", "Image Type"=w80) -> ("New Image"=w106:T2)  [unwired: 3 in, 1 out]
        n46 = call "IMAQ Create"("Image Name"="RaptorTemplate", "Image Type"=w80) -> ("New Image"=w105:T2)  [unwired: 3 in, 1 out]
        n47 = call "IMAQ Create"("Image Name"="Raptor En Face", "Image Type"=w80) -> ("New Image"=w104:T2)  [unwired: 3 in, 1 out]
        n48 = call "create_image_array.vi"("Prefix"="Raptor Fluor Stack" ("Image Name"), "Image Type"=w80, "Num Images"=w91) -> ("Image Array"=w81:T2[])  [unwired: 7 in, 1 out]
        n49 = call "IMAQ Create"("Image Name"="Raptor  Volume En Face", "Image Type"=w80) -> ("New Image"=w100:T2)  [unwired: 3 in, 1 out]
        n50 = call "create_image_array.vi"("Prefix"="Raptor En Face Stack", "Image Type"=w80, "Num Images"=w91) -> ("Image Array"=w102:T2[])  [unwired: 7 in, 1 out]
        n51 = global write "Channel 1 Image Ring.vi" "En Face Image"(w104) -> ()
        n52 = Bundle By Name(cluster=w88, "Current Scan Images"=w97, "Ref Image"=w108, "Ref Cropped"=w107, "Current Image"=w106, "Template"=w105, "En Face"=w104, "En Face Review"=w102, "Volume En Face"=w100, "Fluorescence Review"=w81) -> (w82:T6)
        n53 = Unbundle By Name(w82) -> ("Image Type"=w79:T7)
        n54 = call "IMAQ Create"("Image Name"="Raptor Fluor Line", "Image Type"=w79) -> ("New Image"=w85:T2)  [unwired: 3 in, 1 out]
        n55 = call "IMAQ Create"("Image Name"="Raptor Fluor Image", "Image Type"=w79) -> ("New Image"=w93:T2)  [unwired: 3 in, 1 out]
        n56 = call "IMAQ Create"("Image Name"="Raptor Temp Image", "Image Type"=w79) -> ("New Image"=w83:T2)  [unwired: 3 in, 1 out]
        n57 = call "IMAQ Create"("Image Name"="Raptor Current ROI", "Image Type"=w79) -> ("New Image"=w87:T2)  [unwired: 3 in, 1 out]
        n58 = call "IMAQ Create"("Image Name"="Raptor Ref ROI", "Image Type"=w79) -> ("New Image"=w86:T2)  [unwired: 3 in, 1 out]
        n59 = global write "Channel 2 Image Ring.vi" "Channel 2 Recon"(w93) -> ()
        n60 = Bundle By Name(cluster=w82, "Temp Image"=w83, "Fluorescence Line"=w85, "Fluorescence Image"=w93, "Current ROI"=w87, "Reference ROI"=w86) -> (w95:T6)
      }
      frame "--- PROCESS FLOW ---" {
      }
      frame "wait", Default {
        # "If we are running and we have a frame, queue up\nto process it"
        # "Default state, checks if we are running and have frames to process and if so, queue up 'process image'"
        n61 = Get Queue Status(queue=w117) -> (# elements in queue=w116:i32)  [unwired: 2 in, 7 out]
        "Frame Lag" <- w116
        n62 = Unbundle By Name(w122) -> ("Running"=w118:bool)
        "Running" <- w118
        n63 = Greater Than 0?(x=w116) -> (x > 0?=w121:bool)
        n64 = And(x=w121, y=w118) -> (x .and. y?=w120:bool)
        n65 = case shown="True" w120 {
          tunnel: w119 -> [_ w126]
          frame False {
            n66 = Wait (ms)(milliseconds to wait=u32 1) -> ()  [unwired: 1 out]
          }
          frame True {
            n67 = Enqueue Element(queue=w126, element=raptor_states."process image") -> ()  [unwired: 2 in, 3 out]
          }
        }
      }
      frame "start" {
        # "Starts assembling an en face image."
        n68 = Bundle By Name(cluster=w130, "Running"=TRUE) -> (w128:T6)
      }
      frame "stop" {
        # "Stop assembling an en face image."
        n69 = Bundle By Name(cluster=w133, "Running"=FALSE) -> (w132:T6)
      }
      frame "new scan" {
        # "Clear Volume Reviwe Image"
        # "Clear Fluorescence Image"
        # "Start at centre of top of en face image"
        # "Clear En Face Image"
        # "When we reset the scan, start again from the zeroth\nimage in the ring."
        # "Sets things up for a new en face scan."
        n70 = Enqueue Element(queue=w153, element=raptor_states."start") -> ()  [unwired: 2 in, 3 out]
        n71 = Bundle By Name(cluster=w140, "Line Counter"=0.0, "B Scan Counter"=0.0, "X Pos"=0.0, "Y Pos"=0.0, "Corrected Linepos"=0.0) -> (w147:T6)
        n72 = Unbundle By Name(w147) -> ("Fluorescence Image"=w143:T2, "En Face"=w154:T2, "En Face Width"=w145:i32, "En Face Height"=w144:i32, "Volume En Face"=w150:T2)
        n73 = call "IMAQ SetImageSize"("Y Resolution"=w144, "X Resolution"=w145, "Image"=w154) -> ("Image Out"=w155:T2)  [unwired: 2 in, 1 out]
        n74 = call "IMAQ SetImageSize"("Y Resolution"=w144, "X Resolution"=w145, "Image"=w143) -> ("Image Out"=w142:T2)  [unwired: 2 in, 1 out]
        n75 = call "IMAQ FillImage"("Pixel Value (U8, U16, I16, Float)"=sgl 0.0, "Image"=w155) -> ("Image Out"=w136:T2)  [unwired: 8 in, 1 out]
        n76 = call "IMAQ FillImage"("Pixel Value (U8, U16, I16, Float)"=sgl 0.0, "Image"=w142) -> ("Image Out"=w135:T2)  [unwired: 8 in, 1 out]
        n77 = Initialize Array(T8 {"xPos"=0, "yPos"=0, "B-scan"=0, "Correlation"=0.0, "Frame Step"=0.0} ("Cluster"), w144) -> (w139:T8[])
        n78 = local write "Corrected Fluorescence"(w135) -> ()
        n79 = local write "Corrected En Face"(w136) -> ()
        n80 = call "IMAQ Copy"("Image Dst"=w150, "Image Src"=w136) -> ("Image Dst Out"=w149:T2)  [unwired: 4 in, 1 out]
        n81 = local write "Current Volume En Face Review"(w149) -> ()
        n82 = Bundle By Name(cluster=w147, "Build Record"=w139) -> (w146:T6)
      }
      frame "shutdown" {
        # "Close everything and exit the VI"
      }
      frame "end scan" {
        # "Make the volume review en face \nimage the right size"
        # "Called at the end of a scan. Copies across to en face review (if sufficient lines in en face), sets up volume review size. If continuous scan mode, also sets the new scan to start."
        n83 = Unbundle By Name(w169) -> ("Current Image"=w189:T2)
        n84 = call "IMAQ GetImageSize"("Image"=w189) -> ("Y Resolution"=w188:i32)  [unwired: 3 in, 2 out]
        n85 = Enqueue Element(queue=w166, element=raptor_states."set en face review") -> (queue out=w185:refnum<queue>)  [unwired: 2 in, 2 out]
        n86 = property on="Current Volume Review Selector" class="Slide (strict)"("Scale.Maximum"=w188) -> ()  [unwired: 2 in, 2 out]
        n87 = Unbundle By Name(w169) -> ("Continuous Scan"=w177:bool)
        n88 = Enqueue Element(queue=w185, element=raptor_states."set volume review") -> ()  [unwired: 2 in, 3 out]
        n89 = Enqueue Element(queue=w166, element=raptor_states."generate plots") -> (queue out=w167:refnum<queue>)  [unwired: 2 in, 2 out]
        n90 = Unbundle By Name(w169) -> ("Corrected Linepos"=w164:dbl, "Volume En Face"=w173:T2, "Min Lines for Review"=w175:i32, "Line Counter"=w176:i32, "En Face"=w172:T2, "En Face Review"=w184:T2[], "En Face Counter"=w182:i64, "Num En Face Reviews"=w183:i32, "Fluorescence Image"=w178:T2, "Fluorescence Review"=w179:T2[])
        n91 = case shown="True" w177 {
          tunnel: w167 -> [w206 w208]
          frame False {
            n92 = Enqueue Element(queue=w206, element=raptor_states."stop") -> ()  [unwired: 2 in, 3 out]
          }
          frame True {
            n93 = Enqueue Element(queue=w208, element=raptor_states."new scan") -> ()  [unwired: 2 in, 3 out]
          }
        }
        n94 = call "IMAQ GetImageSize"("Image"=w172) -> ("X Resolution"=w162:i32)  [unwired: 3 in, 2 out]
        n95 = Greater?(x=w176, y=w175) -> (0:w174:bool)
        n96 = Round Toward +Infinity(x=w164) -> (ceil(x): smallest int >= x=w163:dbl)
        n97 = call "IMAQ SetImageSize"("Y Resolution"=w163, "X Resolution"=w162, "Image"=w173) -> ("Image Out"=w171:T2)  [unwired: 2 in, 1 out]
        n98 = call "IMAQ FillImage"("Pixel Value (U8, U16, I16, Float)"=sgl 0.0, "Image"=w171) -> ()  [unwired: 8 in, 2 out]
        n99 = case shown="True" w174 {
          tunnel: w184 -> [_ w204]
          tunnel: w172 -> [_ w198]
          tunnel: w183 -> [_ w203]
          tunnel: w182 -> [w190 w202]
          tunnel: [w190 w201] -> w180
          tunnel: w179 -> [_ w200]
          tunnel: w178 -> [_ w192]
          tunnel: w163 -> [_ w195]
          tunnel: w162 -> [_ w196]
          frame False {
          }
          frame True {
            w194 = 0.0 ("element")
            # "Copy the en face and fluorescence to the review buffer"
            n100 = Increment(x=w202) -> (x+1=w201:i64)
            n101 = Quotient & Remainder(x=w202, y=w203) -> (x-y*floor(x/y)=w199:i64)  [unwired: 1 out]
            n102 = Build Array(w194, w194, w196, w195) -> (w191:dbl[])
            n103 = local write "En Face Review Selector"(w199) -> ()
            n104 = Index Array(array=w204, index=w199) -> (element=w197:T2)
            n105 = Index Array(array=w200, index=w199) -> (element=w193:T2)
            n106 = call "IMAQ Extract 2"("Optional Rectangle"=w191, "Image Dst"=w197, "Image Src"=w198) -> ()  [unwired: 7 in, 2 out]
            n107 = call "IMAQ Extract 2"("Optional Rectangle"=w191, "Image Dst"=w193, "Image Src"=w192) -> ()  [unwired: 7 in, 2 out]
          }
        }
        n108 = Bundle By Name(cluster=w169, "En Face Counter"=w180) -> (w181:T6)
      }
      frame "process image" {
        # "If 1st image then we need to find the surface and prepare\nthe reference ROI now, later this is done by 'handle decorrelation'"
        # "Frame rate calculation"
        # "Grab OCT image from queue"
        # "Grab fluorescence image from queue"
        # "Set in place states to process a new incoming B-scan"
        n109 = Dequeue Element(queue=w233) -> (element=w232:T4)  [unwired: 2 in, 3 out]
        n110 = Unbundle By Name(w213) -> ("B Scan Counter"=w212:i64)
        n111 = Unbundle By Name(w232) -> ("Image"=w226:T2)
        n112 = Equal To 0?(x=w212) -> (x = 0?=w211:bool)
        n113 = case shown="True" w211 {
          tunnel: w218 -> [w234 w239]
          tunnel: [w234 w235] -> w217
          frame False {
          }
          frame True {
            n114 = Enqueue Element(queue=w239, element=raptor_states."surface find") -> (queue out=w237:refnum<queue>)  [unwired: 2 in, 2 out]
            n115 = Enqueue Element(queue=w237, element=raptor_states."prepare reference image") -> (queue out=w235:refnum<queue>)  [unwired: 2 in, 2 out]
          }
        }
        n116 = Unbundle By Name(w213) -> ("Last Line"=w230:dbl, "B Scan Counter"=w216:i64)
        n117 = Unbundle By Name(w213) -> ("Fluorescence Channel"=w222:bool)
        n118 = call <vilib>:"High Resolution Relative Seconds.vi"() -> ("relative seconds"=w229:dbl)
        n119 = Increment(x=w216) -> (x+1=w209:i64)
        "B-scan Processed" <- w209
        n120 = case shown="True" w222 {
          tunnel: w223 -> [_ w242]
          tunnel: [_ w240] -> w221
          frame False {
          }
          frame True {
            n121 = Dequeue Element(queue=w242) -> (element=w241:T4)  [unwired: 2 in, 3 out]
            n122 = Unbundle By Name(w241) -> ("Image"=w240:T2)
          }
        }
        n123 = Subtract(x=w229, y=w230) -> (x-y=w228:dbl)
        n124 = Reciprocal(x=w228) -> (1/x=→"Frame Rate":dbl)
        n125 = Bundle By Name(cluster=w213, "Last Line"=w229, "B Scan Counter"=w209) -> (w225:T6)
        n126 = Enqueue Element(queue=w217, element=raptor_states."shift find") -> (queue out=w220:refnum<queue>)  [unwired: 2 in, 2 out]
        n127 = Enqueue Element(queue=w220, element=raptor_states."check correlation") -> (queue out=w214:refnum<queue>)  [unwired: 2 in, 2 out]
        n128 = Bundle By Name(cluster=w225, "Current Image"=w226, "Fluorescence Line"=w221) -> (w224:T6)
        n129 = Enqueue Element(queue=w214, element=raptor_states."update images") -> ()  [unwired: 2 in, 3 out]
      }
      frame "handle decorrelation" {
        # "Surface finding is slow, so only do not do it every time"
        # "Called if the B scan is sufficently decorrelated, handles adding a line to an image, adding a line to the log, finding the top surface of the next scan, checking the scan is stable (for continuous mode) and checking the en face fits in the image (for auto expand)"
        n130 = Enqueue Element(queue=w247, element=raptor_states."increment linepos") -> (queue out=w261:refnum<queue>)  [unwired: 2 in, 2 out]
        n131 = Unbundle By Name(w251) -> ("Line Counter"=w250:i32, "Surface Find Regularity"=w243:i32)
        n132 = Enqueue Element(queue=w261, element=raptor_states."build corrected OCT") -> (queue out=w258:refnum<queue>)  [unwired: 2 in, 2 out]
        n133 = Quotient & Remainder(x=w250, y=w243) -> (x-y*floor(x/y)=w249:i32)  [unwired: 1 out]
        n134 = Enqueue Element(queue=w258, element=raptor_states."build corrected Fluor") -> (queue out=w246:refnum<queue>)  [unwired: 2 in, 2 out]
        n135 = Equal To 0?(x=w249) -> (x = 0?=w248:bool)
        n136 = Enqueue Element(queue=w246, element=raptor_states."record corrected") -> (queue out=w245:refnum<queue>)  [unwired: 2 in, 2 out]
        n137 = case shown="True" w248 {
          tunnel: w245 -> [w264 w266]
          tunnel: [w264 w265] -> w257
          frame False {
          }
          frame True {
            n138 = Enqueue Element(queue=w266, element=raptor_states."surface find") -> (queue out=w265:refnum<queue>)  [unwired: 2 in, 2 out]
          }
        }
        n139 = Enqueue Element(queue=w257, element=raptor_states."check stable scan") -> (queue out=w253:refnum<queue>)  [unwired: 2 in, 2 out]
        n140 = Enqueue Element(queue=w253, element=raptor_states."prepare reference image") -> (queue out=w254:refnum<queue>)  [unwired: 2 in, 2 out]
        n141 = Unbundle By Name(w251) -> ("Auto Expand"=w255:bool)
        n142 = case shown="True" w255 {
          tunnel: w254 -> [_ w269]
          frame False {
          }
          frame True {
            n143 = Enqueue Element(queue=w269, element=raptor_states."auto expand") -> ()  [unwired: 2 in, 3 out]
          }
        }
      }
      frame "--- DATA FUNCTIONS ---" {
      }
      frame "surface find" {
        # "Make sure depth isn't so deep that we can't pull out a ROI"
        # "Locate the surface line in the current B-scan"
        n144 = case shown="True" TRUE {
          tunnel: w284 -> [w289 w298]
          tunnel: [w288 w297] -> w283
          tunnel: w280 -> [w286 w296]
          tunnel: [w285 w293] -> w279
          frame False {
            n145 = Unbundle By Name(w286) -> ("Current Image"=w291:T2, "Surface Morph SIze"=w290:dbl)  [unwired: 1 out]
            n146 = call "find_surface_simple1.vi"("error in (no error)"=w289, "Filter Size"=w290, "Image In"=w291) -> ("error out"=w288:errorcluster, "surface depth"=w287:dbl)  [unwired: 7 in]
            n147 = Round To Nearest(number=w287) -> (nearest integer value=w285:dbl)
          }
          frame True {
            n148 = Unbundle By Name(w296) -> ("Current Image"=w299:T2, "Surface Morph SIze"=w294:dbl, "Surface Threshold"=w295:dbl)
            n149 = call "find_surface_simple2.vi"("error in"=w298, "Struc El Size"=w294, "Threshold Multiplier"=w295, "Image In"=w299) -> ("error out"=w297:errorcluster, "average surface height"=w292:dbl)  [unwired: 6 in]
            n150 = Round To Nearest(number=w292) -> (nearest integer value=w293:dbl)
          }
        }
        n151 = Unbundle By Name(w280) -> ("ROI Height"=w278:i32, "ROI  Vertical Offset"=w277:i32, "Current Image"=w276:T2)
        n152 = call "IMAQ GetImageSize"("Image"=w276) -> ("Y Resolution"=w274:i32)  [unwired: 3 in, 2 out]
        n153 = Add(x=w278, y=w277) -> (x+y=w275:i32)
        n154 = Subtract(x=w274, y=w275) -> (x-y=w273:i32)
        n155 = Max & Min(x=w273, y=w279) -> (min(x,y)=w272:dbl)  [unwired: 1 out]
        n156 = Bundle By Name(cluster=w280, "Current Depth"=w272) -> (w281:T6)
      }
      frame "shift find" {
        # "Calculates in-plane lateral and axial shift relative to last reference frame by normalised cross correlation"
        n157 = Unbundle By Name(w304) -> ("Current Depth"=w308:i32, "ROI Width"=w310:i32, "ROI Height"=w309:i32, "Vertical Search Range"=w311:i32, "Ref Image"=w312:T2, "Ref Cropped"=w313:T2, "Current Image"=w306:T2, "Template"=w314:T2)
        n158 = call "cross_correlate.vi"("Ref Image Cropped"=w313, "Template Image Cropped"=w314, "Template Height"=w309, "Depth"=w308, "Template Width"=w310, "Vertical Search Range"=w311, "Ref Image"=w312, "Template Image"=w306) -> ("y shift"=w301:i32, "x shift"=w303:i32)  [unwired: 2 out]
        n159 = Negate(x=w303) -> (-x=w302:i32)
        n160 = Negate(x=w301) -> (-x=w300:i32)
        n161 = Bundle By Name(cluster=w304, "X Shift"=w302, "Y Shift"=w300) -> (w307:T6)
      }
      frame "check correlation" {
        # "Correlation between\ncurrent image and\nreference"
        # "Extract ROI from image with shift\napplied"
        # "Mask to exclude bright pixels"
        # "Check to see if current image is decorrelated from reference image. If so, copy current image to reference image and set 'Decorrelated' flag to true so that this line will be added to the enface."
        n162 = Unbundle By Name(w325) -> ("Current Image"=w342:T2, "Current ROI"=w341:T2, "Current Depth"=w340:i32, "ROI  Vertical Offset"=w339:i32, "ROI Width"=w327:i32, "ROI Height"=w326:i32, "X Shift"=w329:i32, "Y Shift"=w331:i32, "Temp Image"=w323:T2, "Mean Filter Size"=w321:i32)
        n163 = Negate(x=w329) -> (-x=w328:i32)
        n164 = Negate(x=w331) -> (-x=w330:i32)
        n165 = Add(x=w340, y=w339) -> (x+y=w334:i32)
        n166 = Unbundle By Name(w325) -> ("Reference Filtered"=w316:dbl[][], "Gaussian Filter Size"=w338:dbl, "Mean Filter Size"=w337:i32)
        n167 = Add(x=w334, y=w330) -> (x+y=w333:i32)
        n168 = call "extract_depth_range_fix_width.vi"("x offset"=w328, "width"=w327, "vertical offset"=w333, "vertical size"=w326, "Image Dst"=w341, "Image"=w342) -> ("Image Dst Out"=w324:T2)  [unwired: 3 in, 2 out]
        n169 = call "speckle_mask.vi"("SE Size"=w321, "Threshold Multiplier"=sgl 5.0, "Image Out"=w323, "Image In"=w324) -> ("Mask Out"=w318:bool[][])  [unwired: 5 in, 2 out]
        n170 = call "pre_filter_image_8bit_dll.vi"("Gaussian Filter Size"=w338, "Mean Filter Size"=w337, "Input Image"=w324) -> ("Output Image Array"=w320:dbl[][])  [unwired: 7 in, 1 out]
        n171 = Not(x=w318) -> (.not. x?=w317:bool[][])
        n172 = call "masked_correlation.vi"("Mask"=w317, "Image 2"=w320, "Image 1"=w316) -> ("correlation coefficient"=w319:dbl)  [unwired: 8 in]
        "Correlation" <- w319
        n173 = Unbundle By Name(w325) -> ("Correlation Thresh"=w336:dbl)
        n174 = Less?(x=w319, y=w336) -> (x < y?=w335:bool)
        "Decorrelated" <- w335
        n175 = Bundle By Name(cluster=w325, "Correlation"=w319) -> (w332:T6)
        n176 = case shown="True" w335 {
          tunnel: w343 -> [_ w344]
          frame False {
          }
          frame True {
            n177 = Enqueue Element(queue=w344, element=raptor_states."handle decorrelation") -> ()  [unwired: 2 in, 3 out]
          }
        }
      }
      frame "prepare reference image" {
        # "Extract and pre-process ROI from reference image"
        n178 = Unbundle By Name(w348) -> ("Current Image"=w351:T2, "Ref Image"=w350:T2, "Reference ROI"=w362:T2, "Current Depth"=w361:i32, "ROI  Vertical Offset"=w360:i32, "ROI Width"=w354:i32, "ROI Height"=w355:i32)
        n179 = Unbundle By Name(w348) -> ("Gaussian Filter Size"=w357:dbl, "Mean Filter Size"=w356:i32)
        n180 = Add(x=w361, y=w360) -> (x+y=w359:i32)
        n181 = call "IMAQ Copy"("Image Dst"=w350, "Image Src"=w351) -> ("Image Dst Out"=w349:T2)  [unwired: 4 in, 1 out]
        n182 = call "extract_depth_range_fix_width.vi"("width"=w354, "vertical offset"=w359, "vertical size"=w355, "Image Dst"=w362, "Image"=w349) -> ("Image Dst Out"=w358:T2)  [unwired: 4 in, 2 out]
        n183 = call "pre_filter_image_8bit_dll.vi"("Gaussian Filter Size"=w357, "error in (no error)"=w352, "Mean Filter Size"=w356, "Input Image"=w358) -> ("error out"=w353:errorcluster, "Output Image Array"=w346:dbl[][])  [unwired: 6 in]
        n184 = Bundle By Name(cluster=w348, "Reference Filtered"=w346) -> (w347:T6)
      }
      frame "build corrected OCT" {
        # "If we moved sufficiently far (i.e. we are decorrelated) add a line from the current B-scan to the en face being assembled."
        n185 = Unbundle By Name(w371) -> ("Current Image"=w369:T2, "En Face"=w370:T2, "X Pos"=w366:i32, "Current Depth"=w363:i32, "Frame Step"=w367:dbl, "Last Line"=w365:dbl, "En Face Depth"=w364:i32, "Track Surface"=w368:bool)
        n186 = call "build_en_face_interp_sequential.vi"("Existing En Face"=w370, "Image to add"=w369, "current x"=w366, "current y"=w363, "depth"=w364, "add height"=w367, "output line"=w365, "Track Surface"=w368) -> ()  [unwired: 11 in, 1 out]
      }
      frame "build corrected Fluor" {
        # "Adds a line to the fluorescence image."
        n187 = Unbundle By Name(w373) -> ("Fluorescence Channel"=w374:bool)
        n188 = disable-structure shown="Enabled" {
          disable-tunnel: w374 -> [w376 _]
          disable-tunnel: w373 -> [w375 _]
          frame Enabled {
            n189 = case shown="True" w376 {
              tunnel: w375 -> [_ w379]
              frame False {
              }
              frame True {
                n190 = Unbundle By Name(w379) -> ("X Pos"=w382:i32, "Fluorescence Image"=w381:T2, "Fluorescence Line"=w380:T2)
                n191 = Unbundle By Name(w379) -> ("Frame Step"=w378:dbl, "Last Line"=w377:dbl)
                n192 = call "add_line_to_enface.vi"("En Face Image"=w381, "Shift"=w382, "Raw Image"=w380, "Add Height"=w378, "Input Line"=0.0, "Output Line"=w377) -> ()  [unwired: 8 in, 2 out]
              }
            }
          }
          frame Disabled {
          }
        }
      }
      frame "record corrected" {
        # "Note - yPos in record is\nthe surface pos from find surface, \nnot the integrated yPos from the\nshifts from the norm xc."
        # "Store a record of where the current line in the en face came from"
        n193 = Unbundle By Name(w387) -> ("Build Record"=w396:T8[], "X Pos"=w398:i32, "B Scan Counter"=w397:i64, "Correlation"=w391:dbl, "Line Counter"=w389:i32, "Current Depth"=w393:i32, "Frame Step"=w390:dbl)  [unwired: 2 out]
        n194 = Unbundle By Name(w387) -> ("Current Image"=w384:T2, "Current Scan Images"=w386:T2[])
        n195 = Decrement(x=w389) -> (x-1=w385:i32)
        n196 = Round To Nearest(number=w393) -> (nearest integer value=w392:i32)
        n197 = Index Array(array=w396, index=w385) -> (element=w399:T8)
        n198 = call "add_to_ring_buffer.vi"("Buffer Position"=w385, "Ring Buffer"=w386, "Image"=w384) -> ()  [unwired: 5 in, 4 out]
        n199 = Bundle By Name(cluster=w399, "xPos"=w398, "yPos"=w392, "B-scan"=w397, "Correlation"=w391, "Frame Step"=w390) -> (w395:T8)
        n200 = Insert Into Array(array=w396, index=w385, new element=w395) -> (w394:T8[])
        n201 = Bundle By Name(cluster=w387, "Build Record"=w394) -> (w400:T6)
      }
      frame "check stable scan" {
        # "If using continuous scan check if scan  is stable (not completely decorrelating between each B-scan) end scan and start another."
        n202 = Unbundle By Name(w402) -> ("Continuous Scan"=w401:bool)
        n203 = case shown="True" w401 {
          tunnel: w403 -> [_ w410]
          tunnel: w402 -> [_ w407]
          frame False {
          }
          frame True {
            n204 = Unbundle By Name(w407) -> ("Stability Length"=w406:i32)
            n205 = Unbundle By Name(w407) -> ("Line Counter"=w409:i32, "Build Record"=w411:T8[])
            n206 = Greater?(x=w409, y=w406) -> (0:w408:bool)
            n207 = case shown="True" w408 {
              tunnel: w411 -> [_ w426]
              tunnel: w406 -> [_ w423]
              tunnel: w409 -> [_ w418]
              tunnel: [_ w412] -> w405
              frame False {
              }
              frame True {
                n208 = Decrement(x=w418) -> (x-1=w417:i32)
                n209 = for {
                  N: w423 -> [_]
                  tunnel: w426 -> [w432]
                  tunnel: w417 -> [w431]
                  tunnel: [w427] -> w419 mode=indexing
                  i -> [w430]
                  n210 = Subtract(x=w431, y=w430) -> (x-y=w429:i32)
                  n211 = Index Array(array=w432, index=w429) -> (element=w428:T8)
                  n212 = Unbundle By Name(w428) -> ("B-scan"=w427:i32)
                }
                n213 = Decrement(x=w423) -> (x-1=w420:i32)
                n214 = Array Subset(array=w419, index=1) -> (w415:i32[])  [unwired: 1 in]
                n215 = Array Subset(array=w419, index=0, length=w420) -> (w416:i32[])
                n216 = Subtract(x=w416, y=w415) -> (x-y=w422:i32[])
                n217 = Add Array Elements(numeric array=w422) -> (sum=w421:i32)
                n218 = Divide(x=w421, y=w420) -> (x/y=w413:dbl)
                n219 = Less Or Equal?(x=w413, y=1.0) -> (x <= y?=w412:bool)
              }
            }
            n220 = case shown="True" w405 {
              tunnel: w410 -> [_ w433]
              frame False {
              }
              frame True {
                n221 = Enqueue Element(queue=w433, element=raptor_states."end scan") -> ()  [unwired: 2 in, 3 out]
              }
            }
          }
        }
      }
      frame "increment linepos" {
        # "Cummulative positions from shifts"
        # "This is the 'interpolation method' - looks how far below\ncorrelation threshold we have gone and calculates a frame step\nwhich is > 1."
        # "Check for maximum size of scan reached"
        # "Start using this surface as a reference"
        # "Moves down the real-time en-face image, incrmenting counters and calculating the 'step' we need to take depending on the estimate velocity."
        n222 = Unbundle By Name(w447) -> ("En Face Height"=w455:i32, "X Shift"=w459:i32, "X Pos"=w457:i32, "Y Shift"=w458:i32, "Y Pos"=w456:i32, "Corrected Linepos"=w435:dbl)
        "Y Shift" <- w458
        "X Shift" <- w459
        "X Position" <- w457
        "Y Position" <- w456
        n223 = Unbundle By Name(w447) -> ("Aspect Ratio"=w438:dbl, "Correlation"=w446:dbl, "Correlation Thresh"=w444:dbl)
        n224 = Unbundle By Name(w447) -> ("Line Counter"=w450:i32)
        n225 = Unbundle By Name(w447) -> ("Current Image"=w462:T2, "Ref Image"=w463:T2)
        n226 = Increment(x=w450) -> (x+1=w448:i32)
        n227 = Subtract(x=w444, y=w446) -> (x-y=w442:dbl)
        n228 = Add(x=w459, y=w457) -> (x+y=w461:i32)
        n229 = Add(x=w458, y=w456) -> (x+y=w460:i32)
        n230 = call "IMAQ Copy"("Image Dst"=w463, "Image Src"=w462) -> ()  [unwired: 4 in, 2 out]
        n231 = Subtract(x=1.0, y=w444) -> (x-y=w441:dbl)
        n232 = Divide(x=w442, y=w441) -> (x/y=w443:dbl)
        n233 = Add(x=w443, y=1.0) -> (x+y=w439:dbl)
        n234 = Multiply(x=w438, y=w439) -> (x*y=w437:dbl)
        "Frame Step" <- w437
        n235 = Add(x=w435, y=w437) -> (x+y=w436:dbl)
        "En Face Line" <- w436
        n236 = Round Toward +Infinity(x=w436) -> ()  [unwired: 1 out]
        n237 = Bundle By Name(cluster=w447, "Frame Step"=w437, "Line Counter"=w448) -> (w449:T6)
        n238 = Bundle By Name(cluster=w449, "X Pos"=w461, "Y Pos"=w460, "Corrected Linepos"=w436, "Last Line"=w435) -> (w451:T6)
        n239 = Greater?(x=w436, y=w455) -> (0:w453:bool)
        n240 = case shown="True" w453 {
          tunnel: w452 -> [_ w465]
          frame False {
          }
          frame True {
            n241 = Enqueue Element(queue=w465, element=raptor_states."end scan") -> ()  [unwired: 2 in, 3 out]
          }
        }
      }
      frame "auto expand" {
        # "Checks if en-face has gone outside the image and if so increases the image sizes for live en face and fluorescence images"
        n242 = Unbundle By Name(w468) -> ("En Face"=w466:T2, "Fluorescence Image"=w467:T2, "X Pos"=w470:i32, "Current Image"=w471:T2)
        n243 = call "check_expand_needed.vi"("Insert Pos"=w470, "Insert Image"=w471, "Larger Image"=w467) -> ("Either"=w469:bool)  [unwired: 5 in, 3 out]
        n244 = case shown="True" w469 {
          tunnel: w468 -> [_ w476]
          tunnel: w467 -> [_ w474]
          tunnel: w466 -> [_ w475]
          frame False {
          }
          frame True {
            n245 = Unbundle By Name(w476) -> ("Expand Step"=w473:i32)
            n246 = call "expand_image_horizontal.vi"("Expand By"=w473, "Image"=w474) -> ()  [unwired: 8 in, 2 out]
            n247 = call "expand_image_horizontal.vi"("Expand By"=w473, "Image"=w475) -> ()  [unwired: 8 in, 2 out]
          }
        }
      }
      frame "--- GUI HANDING ---" {
      }
      frame "update images" {
        # "For speed, do not updates every frame"
        # "Updates image display and call update plots"
        n248 = Unbundle By Name(w485) -> ("B Scan Counter"=w484:i64, "Image Display Regularity"=w480:i32)
        n249 = Quotient & Remainder(x=w484, y=w480) -> (x-y*floor(x/y)=w483:i64)  [unwired: 1 out]
        n250 = Equal To 0?(x=w483) -> (x = 0?=w482:bool)
        n251 = case shown="True" w482 {
          tunnel: w485 -> [_ w488]
          tunnel: w481 -> [_ w487]
          frame False {
          }
          frame True {
            n252 = Unbundle By Name(w488) -> ("Current Image"=→"Current B Scan":T2, "En Face"=→"Corrected En Face":T2, "Fluorescence Image"=→"Corrected Fluorescence":T2)
            n253 = Enqueue Element(queue=w487, element=raptor_states."generate plots") -> ()  [unwired: 2 in, 3 out]
          }
        }
      }
      frame "update parameters" {
        # "Update parameters which can be changed without an initialisation."
        n254 = local read "Enface Display Depth"() -> (w492:i64)
        n255 = Bundle By Name(cluster=w494, "En Face Depth"=w492) -> (w493:T6)
      }
      frame "generate plots" {
        w510 = u16 2 items=["2nd Order Central", "4th Order Central", "Forward", "Backward"] ("method")
        # "Divide by aspect ratio as the\nframe step was multiplied\nby this in increment linepos\nand we want the graph to\nbe in until of decorrelation \ndistance."
        # "Draws plots of positions and velocity"
        n256 = Unbundle By Name(w499) -> ("Build Record"=w511:T8[])
        n257 = for {
          tunnel: w511 -> [w518] mode=indexing
          tunnel: [w517] -> w504 mode=indexing if=w513
          tunnel: [w516] -> w503 mode=indexing if=w513
          tunnel: [w515] -> w495 mode=indexing if=w513
          tunnel: [w514] -> w505 mode=indexing if=w513
          tunnel: [w512] -> _ mode=indexing
          n258 = Unbundle By Name(w518) -> ("Frame Step"=w512:dbl, "B-scan"=w514:i32, "Frame Step"=w515:dbl, "xPos"=w517:i32, "yPos"=w516:i32)
          n259 = Greater Than 0?(x=w514) -> (x > 0?=w513:bool)
        }
        n260 = Array Max & Min(array=w505) -> (max value=w508:i32)  [unwired: 3 out]
        n261 = Bundle(w505, w504) -> (→"Lateral Position":cluster{i32[], i32[]})  [unwired: 1 in]
        n262 = Bundle(w505, w503) -> (→"Surface Position":cluster{i32[], i32[]})  [unwired: 1 in]
        n263 = Build Array(w508) -> (w509:i32[])
        n264 = call <vilib>:"Derivative x(t).vi"("method"=w510, "Final Condition"=w509, "X"=w505) -> ("dX/dt"=w506:dbl[])  [unwired: 7 in, 1 out]
        n265 = Unbundle By Name(w499) -> ("Aspect Ratio"=w497:dbl)
        n266 = Reciprocal(x=w506) -> (1/x=w500:dbl[])
        n267 = Multiply(x=w500, y=w495) -> (x*y=w498:dbl[])
        n268 = Divide(x=w498, y=w497) -> (x/y=w496:dbl[])
        n269 = Bundle(w505, w496) -> (→"Velocity":cluster{i32[], dbl[]})  [unwired: 1 in]
      }
      frame "set en face review" {
        # "Updates the en face and fluorescence image review with the currently selected en face and fluorescence image from the slider"
        n270 = Unbundle By Name(w523) -> ("Fluorescence Review"=w522:T2[], "En Face Review"=w525:T2[])
        n271 = Index Array(array=w525, index="En Face Review Selector") -> (element=→"En Face Review":T2)
        n272 = Index Array(array=w522, index="En Face Review Selector") -> (element=→"Fluorescence Review":T2)
      }
      frame "set volume review" {
        # "Builds a corrected en face at a required depth"
        n273 = Unbundle By Name(w532) -> ("Volume Review Depth Shown"=w530:i64, "Current Scan Images"=w534:T2[], "Build Record"=w533:T8[], "Volume En Face"=w535:T2)
        n274 = Not Equal?(x="Current Volume Review Selector", y=w530) -> (x != y?=w528:bool)
        n275 = case shown="True" w528 {
          tunnel: w535 -> [_ w542]
          tunnel: w534 -> [_ w540]
          tunnel: w533 -> [_ w539]
          tunnel: "Current Volume Review Selector" -> [w536 w537]
          tunnel: [w536 w537] -> w527
          frame False {
          }
          frame True {
            n276 = call "raptor_build_enface.vi"("Track Surface"="Track Surface", "Depth"=w537, "Volume En Face In"=w542, "Build Record"=w539, "B Scans"=w540) -> ("Volume En Face Out"=→"Current Volume En Face Review":T2)  [unwired: 5 in, 1 out]
          }
        }
        n277 = Bundle By Name(cluster=w532, "Volume Review Depth Shown"=w527) -> (w531:T6)
      }
      frame "--- LOAD AND SAVE ---" {
      }
      frame "save all" {
        # "Saves both en face and fluorescence"
        n278 = Enqueue Element(queue=w549, element=raptor_states."save en face") -> (queue out=w548:refnum<queue>)  [unwired: 2 in, 2 out]
        n279 = Enqueue Element(queue=w548, element=raptor_states."save fluorescence") -> ()  [unwired: 2 in, 3 out]
      }
      frame "save en face" {
        # "Saves the en face currently displayed in the en face review"
        n280 = local read "En Face Review Selector"() -> (w553:i8)
        n281 = Unbundle By Name(w558) -> ("En Face Review"=w557:T2[])
        n282 = Index Array(array=w557, index=w553) -> (element=w556:T2)
        n283 = call "get_filename_from_timestamp.vi"("Suffix"="_en face", "Path"="Save Folder") -> ("Tif"=w554:path)  [unwired: 7 in, 2 out]
        n284 = call-poly "IMAQ Write File 2"("File Path"=w554, "Image"=w556) -> ()  [unwired: 8 in, 2 out]
      }
      frame "save fluorescence" {
        # "Saves the fluorescence iamges currently displayed in the fluorescence review"
        n285 = Unbundle By Name(w561) -> ("Fluorescence Channel"=w560:bool)
        n286 = case shown="True" w560 {
          tunnel: w561 -> [_ w566]
          frame False {
          }
          frame True {
            n287 = local read "En Face Review Selector"() -> (w564:i8)
            n288 = Unbundle By Name(w566) -> ("Fluorescence Review"=w565:T2[])
            n289 = Index Array(array=w565, index=w564) -> (element=w568:T2)
            n290 = local read "Save Folder"() -> (w563:path)
            n291 = call "get_filename_from_timestamp.vi"("Suffix"="_fluor", "Path"=w563) -> ("Tif"=w567:path)  [unwired: 7 in, 2 out]
            n292 = call-poly "IMAQ Write File 2"("File Path"=w567, "Image"=w568) -> ()  [unwired: 8 in, 2 out]
          }
        }
      }
      frame "save volume" {
        # "Saves all the B-Scans recorded to an binary data file"
        n293 = Unbundle By Name(w573) -> ("Current Scan Images"=w583:T2[])
        n294 = Unbundle By Name(w573) -> ("Fluorescence Image"=w575:T2)
        n295 = Unbundle By Name(w573) -> ("Line Counter"=w569:i32)
        n296 = local read "Save Folder"() -> (w590:path)
        n297 = call "get_filename_from_timestamp.vi"("Suffix"="_vol", "Path"=w590) -> ("Tif"=w574:path, "Bin"=w588:path)  [unwired: 7 in, 1 out]
        n298 = Index Array(array=w583, index=0) -> (element=w579:T2)
        n299 = call-poly "IMAQ Write File 2"("File Path"=w574, "Image"=w575) -> ()  [unwired: 8 in, 2 out]
        n300 = call "img_open_file.vi"("error in"=w572, "Operation (open)"=enum16{"Open", "Create/Replace"}."Create/Replace", "Filename"=w588) -> ("error out"=w586:errorcluster, "lpBytesPerSector"=w578:u32, "hFile"=w585:i64)  [unwired: 5 in, 1 out]
        n301 = call "IMAQ GetImageSize"("Image"=w579) -> ("Y Resolution"=w580:i32, "X Resolution"=w581:i32)  [unwired: 3 in, 1 out]
        n302 = call "img_write_file_header.vi"("Y count"=w580, "X count"=w581, "Frame Count"=w569, "error in"=w586, "sector size (512)"=w578, "Image In"=w579, "hFile"=w585) -> ("error out"=w577:errorcluster, "hFile out"=w584:i64)  [unwired: 1 in, 2 out]
        n303 = for {
          N: w569 -> [w594]
          tunnel: w583 -> [w598] mode=indexing
          tunnel: w584 -> [w600]
          tunnel: w578 -> [w599]
          tunnel: [w596] -> w576
          shift-right: [w591] -> w571
          shift-left: w577 -> [w597]
          i -> [w595]
          n304 = call "img_write_image.vi"("error in"=w597, "Sector size (512)"=w599, "Image In"=w598, "hFile"=w600) -> ("error out"=w592:errorcluster, "hFile out"=w596:i64)  [unwired: 4 in, 2 out]
          n305 = call "For Loop Progress Bar.vi"("Message"="Saving", "Total Iter"=w594, "error in (no error)"=w592, "Current Iter"=w595) -> ("error out"=w591:errorcluster)  [unwired: 7 in]
        }
        n306 = call "img_close_file.vi"("error in"=w571, "hFile"=w576) -> ("error out"=w570:errorcluster)  [unwired: 9 in]
      }
      frame "save volume en face" {
        # "Saves the currently visible en face from the volume"
        n307 = local read "Current Volume Review Selector"() -> (w602:i64)
        n308 = Unbundle By Name(w605) -> ("Volume En Face"=w606:T2)
        n309 = Number To Decimal String(number=w602) -> (decimal integer string=w603:string)  [unwired: 1 in]
        n310 = Concatenate Strings("_En Face Depth_" ("Suffix"), w603) -> (w601:string)
        n311 = local read "Save Folder"() -> (w609:path)
        n312 = call "get_filename_from_timestamp.vi"("Suffix"=w601, "Path"=w609) -> ("Tif"=w610:path)  [unwired: 7 in, 2 out]
        n313 = call-poly "IMAQ Write File 2"("error in (no error)"=w608, "File Path"=w610, "Image"=w606) -> ("error out"=w607:errorcluster)  [unwired: 7 in, 1 out]
      }
    }
  }
  n314 = while {
    tunnel: w4 -> [w612]
    tunnel: w14 -> [w618]
    stop <- w615 stop-if-true
    # "Event and Message Handler"
    n315 = Dequeue Element(queue=w618, timeout in ms (-1)=1) -> (element=w616:T5, timed out?=w617:bool)  [unwired: 1 in, 2 out]
    n316 = case shown="False" w617 {
      tunnel: w616 -> [w624 _]
      tunnel: w612 -> [w622 _]
      tunnel: [w621 _] -> w613
      frame False {
        # "We have some message, so process it."
        n317 = Unbundle By Name(w624) -> ("Message"=w623:T9, "Data"=w620:variant)
        n318 = case shown="\"set depth\"" w623 {
          tunnel: w622 -> [w626 w627 w629 w631 w640 w642 w644]
          tunnel: [_ _ _ TRUE _ _ _] -> w621
          tunnel: w620 -> [_ _ _ _ w638 _ _]
          frame "start", Default {
            n319 = Enqueue Element(queue=w626, element=raptor_states."start") -> ()  [unwired: 2 in, 3 out]
          }
          frame "stop" {
            n320 = Enqueue Element(queue=w627, element=raptor_states."stop") -> ()  [unwired: 2 in, 3 out]
          }
          frame "initialise" {
            n321 = Enqueue Element(queue=w629, element=raptor_states."initialise") -> ()  [unwired: 2 in, 3 out]
          }
          frame "shutdown" {
            n322 = Enqueue Element(queue=w631, element=raptor_states."shutdown") -> ()  [unwired: 2 in, 3 out]
          }
          frame "set depth" {
            n323 = Variant To Data(type=0, Variant=w638) -> (data=w636:i32)  [unwired: 1 in, 1 out]
            n324 = local read "Raptor Parameters"() -> (w635:T1)
            n325 = Bundle By Name(cluster=w635, "En Face Depth"=w636) -> (w634:T1)
            n326 = local write "Raptor Parameters"(w634) -> ()
            n327 = Enqueue Element(queue=w640, element=raptor_states."update parameters") -> ()  [unwired: 2 in, 3 out]
          }
          frame "new scan" {
            n328 = Enqueue Element(queue=w642, element=raptor_states."new scan") -> ()  [unwired: 2 in, 3 out]
          }
          frame "end scan" {
            n329 = Enqueue Element(queue=w644, element=raptor_states."end scan") -> ()  [unwired: 2 in, 3 out]
          }
        }
      }
      frame True {
      }
    }
    n330 = event shown="[11] \"New Scan Button\": Value Change" {
      selector: _ -> [_ _ _ _ _ _ _ _ _ _ _ _]
      dyn-events: _ -> [_ _ _ _ _ _ _ _ _ _ _ _]
      timeout: 1 -> [_ _ _ _ _ _ _ _ _ _ _ _]
      tunnel: [_ TRUE _ _ _ _ _ _ _ _ _ _] -> w614
      tunnel: w612 -> [_ w646 w650 w651 w654 w658 w660 w663 w665 w668 w671 _]
      event Timeout {
        n331 = event-data() -> ()  [unwired: 1 in, 3 out]
      }
      event "Shutdown Button": Value Change {
        n332 = event-data() -> ()  [unwired: 1 in, 6 out]
        n333 = local write "Shutdown Button"(FALSE ("Shutdown Button")) -> ()
        n334 = Enqueue Element(queue=w646, element=raptor_states."shutdown") -> ()  [unwired: 2 in, 3 out]
      }
      event "Enface Display Depth": Value Change {
        n335 = event-data() -> ()  [unwired: 1 in, 6 out]
        n336 = Enqueue Element(queue=w650, element=raptor_states."update parameters") -> ()  [unwired: 2 in, 3 out]
      }
      event "Stop Button": Value Change {
        n337 = event-data() -> ()  [unwired: 1 in, 6 out]
        n338 = local write "Stop Button"(FALSE ("Stop Button")) -> ()
        n339 = Enqueue Element(queue=w651, element=raptor_states."stop") -> ()  [unwired: 2 in, 3 out]
      }
      event "Start Button": Value Change {
        n340 = event-data() -> ()  [unwired: 1 in, 6 out]
        n341 = local write "Start Button"(FALSE ("Stop Button")) -> ()
        n342 = Enqueue Element(queue=w654, element=raptor_states."start") -> ()  [unwired: 2 in, 3 out]
      }
      event "En Face Review Selector": Value Change {
        n343 = event-data() -> ()  [unwired: 1 in, 6 out]
        n344 = Enqueue Element(queue=w658, element=raptor_states."set en face review") -> ()  [unwired: 2 in, 3 out]
      }
      event "Current Volume Review Selector": Value Change {
        n345 = event-data() -> ()  [unwired: 1 in, 6 out]
        n346 = Enqueue Element(queue=w660, element=raptor_states."set volume review") -> ()  [unwired: 2 in, 3 out]
      }
      event "Save En Face Button": Value Change {
        n347 = event-data() -> ()  [unwired: 1 in, 6 out]
        n348 = local write "Save En Face Button"(FALSE ("Save En Face Button")) -> ()
        n349 = Enqueue Element(queue=w663, element=raptor_states."save all") -> ()  [unwired: 2 in, 3 out]
      }
      event "Track Surface": Value Change {
        n350 = event-data() -> ()  [unwired: 1 in, 6 out]
        n351 = Enqueue Element(queue=w665, element=raptor_states."set volume review") -> ()  [unwired: 2 in, 3 out]
      }
      event "Save En Face From Volume": Value Change {
        n352 = event-data() -> ()  [unwired: 1 in, 6 out]
        n353 = local write "Save En Face From Volume"(FALSE ("Save En Face From Volume")) -> ()
        n354 = Enqueue Element(queue=w668, element=raptor_states."save volume en face") -> ()  [unwired: 2 in, 3 out]
      }
      event "Save Volume Button": Value Change {
        n355 = event-data() -> ()  [unwired: 1 in, 6 out]
        n356 = local write "Save Volume Button"(FALSE ("Save Volume Button")) -> ()
        n357 = Enqueue Element(queue=w671, element=raptor_states."save volume") -> ()  [unwired: 2 in, 3 out]
      }
      event "New Scan Button": Value Change {
        n358 = event-data() -> ()  [unwired: 1 in, 6 out]
        n359 = local write "New Scan Button"(FALSE ("New Scan Button")) -> ()
        n360 = call "raptor_initialise.vi"() -> ()  [unwired: 11 in, 1 out]
      }
    }
    n361 = Or(x=w614, y=w613) -> (x .or. y?=w615:bool)
  }
